vi "H2O_DIAL_NCAR_4CH_v4.04.vi"() -> ()   [LabVIEW 2012]
uses:
  C:/Users/H2ODial/Desktop/Shared Telescope WV DIAL Code/Libraries and VIs/PowerMeterCommands.dll
  Libraries and VIs/PowerMeterCommands.dll
  <vilib>/DAQmx/write.llb/DAQmx Write (Digital 1D Bool NChan 1Samp 1Line).vi
  <vilib>/DAQmx/miscellaneous.llb/DAQmx Fill In Error Info.vi
  <vilib>/Analysis/baseanly.llb/Mean (DBL).vi
  Libraries and VIs/Scalar_Data.vi
  Libraries and VIs/Scalar_Data_3.vi
  Libraries and VIs/Scalar_Data_2.vi
  Libraries and VIs/Scalar_Data_4.vi
  <vilib>/Analysis/NI_AALBase.lvlib
  Libraries and VIs/CLDevIFace.dll
panel:
  out "FileHour":i32=19
  out "L_Count":i32=64
  out "sigma_off_total":dbl[](array[numeric])=[5.235525125067343e-25, 5.206358319245337e-25, 5.177318750524933e-25, 5.148406424862825e-25, 5.119621341127451e-25, 5.090963491196627e-25, 5.062432860011865e-25, 5.034029425635027e-25, 5.005753159352157e-25, 4.977604025706667e-25, 4.949581982592347e-25, 4.921686981325722e-25, 4.893918966711095e-25, 4.866277877122191e-25, 4.8387636445644285e-25, 4.811376194764721e-25, 4.784115447230487e-25, 4.756981315339233e-25, 4.729973706394386e-25, 4.703092521721628e-25, 4.6763376567211625e-25, 4.6497090009594435e-25, 4.623206438225019e-25, 4.596829846622293e-25, 4.57057909862005e-25, 4.544454061150213e-25, 4.518454595652437e-25, 4.492580558158126e-25, 4.4668317993693425e-25, 4.441208164702635e-25, 4.41570949437918e-25, 4.390335623482575e-25, 4.365086382028137e-25, 4.339961595028071e-25, 4.314961082547237e-25, 4.290084659777996e-25, 4.2653321370993085e-25, 4.240703320135042e-25, 4.216198009811418e-25, 4.191816002426457e-25, 4.16755708969195e-25, 4.143421058805604e-25, 4.1194076924960845e-25, 4.095516769084665e-25, 4.0717480625238245e-25, 4.0481013424706545e-25, 4.0245763743206737e-25, 4.001172919260011e-25, 3.977890734322512e-25, 3.9547295724256756e-25, 3.931689182419048e-25, 3.908769309139365e-25, 3.8859696934393876e-25, 3.863290072236815e-25, 3.840730178557474e-25, 3.8182897415734565e-25, 3.7959684866403156e-25, 3.773766135338825e-25, 3.7516824055099053e-25, 3.729717011286995e-25, 3.707869663137923e-25, 3.686140067893342e-25, 3.664527928779591e-25, 3.643032945453827e-25, 3.621654814033011e-25, 3.600393227122229e-25, 3.579247873843723e-25, 3.5582184398664743e-25, 3.5373046074361216e-25, 3.5165060553938904e-25, 3.4958224592064764e-25, 3.475253490990589e-25, 3.454798819536632e-25, 3.4344581103303625e-25, 3.414231025576395e-25, 3.394117224218377e-25, 3.37411636196096e-25, 3.3542280912885406e-25, 3.3344520614845767e-25, 3.3147879186525413e-25, 3.295235305730259e-25, 3.275793862509532e-25, 3.2564632256504646e-25, 3.237243028702917e-25, 3.2181329021119735e-25, 3.1991324732434905e-25, 3.180241366390581e-25, 3.161459202790299e-25, 3.142785600633377e-25, 3.1242201750825597e-25, 3.1057625382770893e-25, 3.0874122993477767e-25, 3.0691690644282785e-25, 3.051032436660927e-25, 3.0330020162078266e-25, 3.0150774002602592e-25, 2.997258183045521e-25, 2.979543955833093e-25, 2.961934306943937e-25, 2.944428821752431e-25, 2.9270270826932477e-25, 2.909728669267514e-25, 2.8925331580414936e-25, 2.875440122654977e-25, 2.8584491338173137e-25, 2.841559759313169e-25, 2.8247715639976386e-25, 2.80808410980223e-25, 2.791496955724979e-25, 2.775009657833479e-25, 2.7586217692567447e-25, 2.742332840183121e-25, 2.7261424178518227e-25, 2.710050046547509e-25, 2.6940552675881075e-25, 2.6781576193155516e-25, 2.6623566370876434e-25, 2.646651853260364e-25, 2.6310427971768174e-25, 2.615528995144771e-25, 2.600109970428841e-25, 2.5847852432207883e-25, 2.569554330624564e-25, 2.554416746633416e-25, 2.5393720020962457e-25, 2.5244196047033826e-25, 2.5095590589459477e-25, 2.4947898660936654e-25, 2.480111524155541e-25, 2.4655235278440513e-25, 2.451025368544176e-25, 2.436616534266772e-25, 2.422296509605852e-25, 2.408064775697375e-25, 2.3939208101763006e-25, 2.3798640871112015e-25, 2.365894076971971e-25, 2.352010246556833e-25, 2.3382120589521406e-25, 2.324498973455175e-25, 2.3108704455300754e-25, 2.2973259267270024e-25, 2.283864864626908e-25, 2.270486702764721e-25, 2.257190880557015e-25, 2.2439768332388837e-25, 2.2308439917739663e-25, 2.2177917827749597e-25, 2.20481962844103e-25, 2.19192694645104e-25, 2.179113149897461e-25, 2.166377647190967e-25, 2.153719841983278e-25, 2.1411391330535246e-25, 2.1286349142540036e-25, 2.1162065743868337e-25, 2.103853497130775e-25, 2.091575060946101e-25, 2.079370638983031e-25, 2.0672395989815037e-25, 2.0551813031976677e-25, 2.0431951082869756e-25, 2.0312803652523447e-25, 2.019436419319984e-25, 2.0076626098781596e-25, 1.9959582703908636e-25, 1.9843227283026113e-25, 1.9727553050009988e-25, 1.9612553156963306e-25, 1.9498220693936616e-25, 1.9384548688025462e-25, 1.9271530103114487e-25, 1.915915783921294e-25, 1.9047424731896738e-25, 1.8936323552292957e-25, 1.8825847006561212e-25, 1.8715987735714719e-25, 1.8606738315918164e-25, 1.8498091257941087e-25, 1.8390039007904753e-25, 1.8282573946936752e-25, 1.8175688392200846e-25, 1.80693745969556e-25, 1.7963624751388698e-25, 1.7858430983630522e-25, 1.7753785360393623e-25, 1.7649679888396773e-25, 1.7546106515613228e-25, 1.7443057132789558e-25, 1.7340523575155863e-25, 1.723849762422857e-25, 1.7136971010131167e-25, 1.7035935413825008e-25, 1.6935382469544605e-25, 1.6835303767796407e-25, 1.6735690858143057e-25, 1.6636535252563445e-25, 1.653782842907513e-25, 1.643956183497921e-25, 1.6341726891478545e-25, 1.624431499756322e-25, 1.6147317534796005e-25, 1.6050725871551994e-25, 1.5954531368896971e-25, 1.585872538492723e-25, 1.576329928151117e-25, 1.566824442883223e-25, 1.5573552212546758e-25, 1.5479214039898043e-25, 1.5385221346219397e-25, 1.5291565602013113e-25, 1.519823831962039e-25, 1.5105231061650234e-25, 1.5012535447460145e-25, 1.49201431624485e-25, 1.482804596459418e-25, 1.4736235693849326e-25, 1.46447042805166e-25, 1.455344375360034e-25, 1.4462446250285657e-25, 1.4371704024629248e-25, 1.4281209456557682e-25, 1.4190955061389853e-25, 1.410093350012645e-25, 1.4011137586880333e-25, 1.3921560301221658e-25, 1.3832194795253431e-25, 1.3743034404767374e-25, 1.3654072658699072e-25, 1.3565303288298996e-25, 1.3476720236918642e-25, 1.3388317669734332e-25, 1.3300089982893968e-25, 1.3212031812258562e-25, 1.3124138043688156e-25, 1.3036403820696332e-25, 1.2948824553577423e-25, 1.2861395928315612e-25, 1.2774113913410786e-25, 1.2686974768684636e-25, 1.2599975053009544e-25, 1.2513111630057894e-25, 1.2426381676023619e-25, 1.2339782685325752e-25, 1.2253312476934588e-25, 1.2166969199403071e-25, 1.2080751335374065e-25, 1.1994657705541538e-25, 1.1908687474046665e-25, 1.182284014933639e-25, 1.1737115587808914e-25, 1.1651513996305814e-25, 1.1566035931942852e-25, 1.1480682304187532e-25, 1.1395454373665928e-25, 1.1310353751750977e-25, 1.1225382399779688e-25, 1.1140542626706877e-25, 1.1055837085176348e-25, 1.097126877076807e-25, 1.0886841014622313e-25, 1.0802557481625692e-25, 1.07184221622742e-25, 1.0634439369229237e-25, 1.0550613727868173e-25, 1.0466950171251473e-25, 1.038345393031225e-25, 1.0300130526116006e-25, 1.0216985760646603e-25, 1.0134025706453978e-25, 1.0051256696943142e-25, 9.968685315566847e-26, 9.886318383691271e-26, 9.804162950309608e-26, 9.722226278487634e-26, 9.640515833439737e-26, 9.559039270504641e-26]
  out "sigma_on_total":dbl[](array[numeric])=[2.797932674537263e-23, 2.7919260210529697e-23, 2.7857624681005274e-23, 2.7794434391305526e-23, 2.772970398522555e-23, 2.766344851030676e-23, 2.75956834067003e-23, 2.752642449576685e-23, 2.7455687974466073e-23, 2.738349040027496e-23, 2.730984868354913e-23, 2.723478007699131e-23, 2.715830216384083e-23, 2.708043284811922e-23, 2.700119034195852e-23, 2.6920593156696255e-23, 2.683866008939376e-23, 2.675541021372197e-23, 2.6670862865706313e-23, 2.6585037635576785e-23, 2.649795435279164e-23, 2.6409633077211456e-23, 2.632009408457337e-23, 2.622935785817294e-23, 2.613744507314058e-23, 2.6044376589247666e-23, 2.5950173434598757e-23, 2.5854856796179397e-23, 2.5758448009875033e-23, 2.5660968544222956e-23, 2.556243999280564e-23, 2.5462884060976083e-23, 2.5362322554945982e-23, 2.5260777370381022e-23, 2.5158270479358892e-23, 2.505482392145547e-23, 2.4950459792064817e-23, 2.484520023083591e-23, 2.4739067410236316e-23, 2.4632083527131388e-23, 2.452427078874796e-23, 2.4415651405700084e-23, 2.4306247579414987e-23, 2.419608149375398e-23, 2.4085175301631292e-23, 2.397355112043402e-23, 2.3861231018430063e-23, 2.3748237005968667e-23, 2.3634591028590494e-23, 2.352031495518178e-23, 2.3405430569776974e-23, 2.3289959565846446e-23, 2.3173923533947887e-23, 2.3057343955308516e-23, 2.2940242194478666e-23, 2.282263949107109e-23, 2.2704556951731608e-23, 2.258601554403489e-23, 2.2467036088909498e-23, 2.2347639252740327e-23, 2.2227845543076132e-23, 2.2107675300632033e-23, 2.1987148693219933e-23, 2.18662857110243e-23, 2.1745106160433166e-23, 2.162362965811164e-23, 2.1501875625868626e-23, 2.137986328630551e-23, 2.1257611659233766e-23, 2.113513955448302e-23, 2.1012465569339107e-23, 2.0889608084552326e-23, 2.076658526056973e-23, 2.0643415033451598e-23, 2.0520115112091644e-23, 2.0396702974574623e-23, 2.0273195865824679e-23, 2.014961079439288e-23, 2.0025964529993626e-23, 1.9902273602298353e-23, 1.9778554297286174e-23, 1.9654822656439602e-23, 1.9531094474030767e-23, 1.9407385298246202e-23, 1.9283710425220375e-23, 1.916008490311647e-23, 1.9036523527571788e-23, 1.891304084249504e-23, 1.878965113795808e-23, 1.8666368452826158e-23, 1.854320657095235e-23, 1.842017902311335e-23, 1.829729908755202e-23, 1.81745797881863e-23, 1.8052033895967212e-23, 1.7929673929858462e-23, 1.7807512156964232e-23, 1.7685560592802502e-23, 1.756383100364305e-23, 1.744233490557376e-23, 1.732108356659952e-23, 1.7200088008822495e-23, 1.7079359007408066e-23, 1.6958907094876615e-23, 1.6838742559821464e-23, 1.6718875450901883e-23, 1.65993155762526e-23, 1.6480072508541525e-23, 1.6361155583187127e-23, 1.6242573903102193e-23, 1.6124336338929427e-23, 1.600645153253371e-23, 1.5888927898296925e-23, 1.5771773626269717e-23, 1.5654996683162563e-23, 1.553860481518072e-23, 1.5422605551758425e-23, 1.5307006206288193e-23, 1.519181387994595e-23, 1.50770354621203e-23, 1.4962677636431785e-23, 1.4848746879968784e-23, 1.4735249468084555e-23, 1.462219147707836e-23, 1.4509578784447202e-23, 1.439741707535912e-23, 1.4285711842133102e-23, 1.4174468389483338e-23, 1.4063691835697543e-23, 1.3953387115476105e-23, 1.3843558984350844e-23, 1.3734212019927912e-23, 1.3625350624750627e-23, 1.3516979029933517e-23, 1.340910129876358e-23, 1.3301721326484853e-23, 1.3194842846972786e-23, 1.308846943215553e-23, 1.298260449786731e-23, 1.2877251303686642e-23, 1.2772412958726839e-23, 1.2668092421859013e-23, 1.2564292506343541e-23, 1.2461015881516254e-23, 1.2358265075568203e-23, 1.2256042479710005e-23, 1.2154350349122617e-23, 1.2053190805695919e-23, 1.195256584279949e-23, 1.1852477325180829e-23, 1.1752926993686362e-23, 1.1653916466854379e-23, 1.1555447244520414e-23, 1.1457520708062173e-23, 1.1360138126272996e-23, 1.1263300654904525e-23, 1.1167009340815523e-23, 1.1071265124104599e-23, 1.0976068840545527e-23, 1.0881421223367986e-23, 1.0787322906900863e-23, 1.0693774427047456e-23, 1.0600776226092928e-23, 1.0508328652518817e-23, 1.0416431964807624e-23, 1.032508633335529e-23, 1.0234291841778234e-23, 1.014404849115549e-23, 1.0054356199498731e-23, 9.965214805919994e-24, 9.876624071246281e-24, 9.788583681497812e-24, 9.701093249022246e-24, 9.61415231391845e-24, 9.527760347380011e-24, 9.441916752482458e-24, 9.356620866076204e-24, 9.27187196198394e-24, 9.1876692506485e-24, 9.104011883065926e-24, 9.020898950407833e-24, 8.938329487852217e-24, 8.856302474691644e-24, 8.77481683652038e-24, 8.69387144736208e-24, 8.613465130247208e-24, 8.533596659539215e-24, 8.454264762212557e-24, 8.375468119356111e-24, 8.297205367646391e-24, 8.219475100553976e-24, 8.14227587023874e-24, 8.065606188690859e-24, 7.9894645288563e-24, 7.913849326432266e-24, 7.838758980703018e-24, 7.764191856046392e-24, 7.69014628339956e-24, 7.61662056058579e-24, 7.543612954624664e-24, 7.471121702227356e-24, 7.399145011371256e-24, 7.327681061555103e-24, 7.256728006172217e-24, 7.18628397208889e-24, 7.116347062363852e-24, 7.046915355389474e-24, 6.977986907338961e-24, 6.909559752711582e-24, 6.84163190507593e-24, 6.774201358193111e-24, 6.707266086331618e-24, 6.640824046318606e-24, 6.5748731770349155e-24, 6.509411401784767e-24, 6.444436627394219e-24, 6.37994674615007e-24, 6.315939636375851e-24, 6.252413162819167e-24, 6.189365177933176e-24, 6.126793522223083e-24, 6.064696024770319e-24, 6.003070504094802e-24, 5.9419147695012916e-24, 5.8812266199939874e-24, 5.821003847135055e-24, 5.761244233601571e-24, 5.7019455549703875e-24, 5.6431055801137746e-24, 5.584722071428577e-24, 5.526792785547098e-24, 5.469315474021976e-24, 5.41228788367443e-24, 5.3557077567834e-24, 5.299572832346729e-24, 5.243880845770717e-24, 5.188629529638899e-24, 5.133816614447439e-24, 5.079439828285976e-24, 5.0254968978526986e-24, 4.971985548989939e-24, 4.918903506350013e-24, 4.866248494353352e-24, 4.814018237267727e-24, 4.762210459841147e-24, 4.710822887499211e-24, 4.6598532465403046e-24, 4.609299264328646e-24, 4.559158670401048e-24, 4.5094291956991564e-24, 4.460108573396636e-24, 4.4111945394283046e-24, 4.362684832116821e-24, 4.3145771930692756e-24, 4.266869366921456e-24, 4.219559101711097e-24, 4.1726441493533976e-24, 4.1261222657367405e-24, 4.0799912104676045e-24, 4.034248748141451e-24, 3.988892647248926e-24, 3.9439206815329655e-24, 3.899330629138496e-24, 3.8551202738110765e-24, 3.811287404055379e-24, 3.7678298141883e-24, 3.7247453038325186e-24, 3.682031678396438e-24, 3.639686749212774e-24, 3.597708333465123e-24, 3.5560942545295516e-24, 3.514842342094612e-24, 3.473950431977779e-24, 3.4334163667422104e-24, 3.393237995303275e-24, 3.353413173235189e-24, 3.313939763152937e-24]
  out "background start":u32=269
  in  "Tab Control 2":enum32{"WV ND far", "WV ND near"}(tab)
  out "Water Vapor Number Density":dbl[][](graph)=[[2.0850030204725254, 1.6437816356735586, 1.585155342040526, 1.4766994515960457, 1.30036312748755, 1.2199808815388116, 1.2370910084987519, 1.215025732560631, 1.2094080739137962, 1.241574717944049, 1.2400023005883922, 1.27849779833147, 1.1795592586311967, 1.0177397521499008, 0.9252100877503859, 0.7984582340031915, 0.7980739516878171, 0.981563170106793, 1.1781709472616928, 1.2604407853067179, 1.2878310718082464, 0.9634305882669428, 0.6969286050839552, 1.1038803104348858, 1.3635527853492146, 1.2756168466381246, 1.126651831817223, 0.8778144411805149, 1.0190755684005814, 0.7047223129802344, -0.11061275401062327, 0.32290982101144, 0.00359197927144264, -0.7090099831195374, 0.893795498062288, 1.3190587788482702, 0.5035252151885548, 0.28968410009682993, 0.18512581697537367, 0.3528560626576347, 3.2334978562537446, 2.5390776007956823, -0.7673398002393842, -0.394060585705837, 0.1936892729399504, -0.00042004503324332, 0.6488032887854288, -1.7199954662418278, -2.7250956673421256, -2.829602242413674, -2.8562819886715487, 0.24819172415081983, 2.4357247968367557, -0.08684114825213345, 0.33472910263403344, 1.4525262638352578, 0.6864828027636564, -0.8773873676446362, -0.7748026661236419, -0.8964337587498109, -1.3574906833153229, -1.9055460673602915, -1.8292121536809087, -2.635674405161918, -4.437757131889345, -5.4711270091092965, -4.930064996443606, -2.073930252529242, -0.56696116876414, 3.0237519462406395, 4.188864159369365, -1.179054090698212, -2.0895392573583993, 1.096562317594488, 3.8376615661152935, 3.813963625998703, 4.150238128596571, 1.2755121222242172, 1.722039359608823, -5.434206523456943, -5.690067282284008, 0.05770429680683136, 0.2219851428874463, 7.0959946213841985, 1.532667826481585, -0.5776567177838131, -3.1758034812173244, 3.496673290983224, 0.04729286306369408, 0.19208777119169312, 4.302023971326133, 0.01865185774192832, 1.2460870798892005, -2.484809490618561, -0.6929405246784887, 1.5500192808793258, -0.05367189562925824, -5.735849575728608, -10.29033614959377, -6.410256857872558, -5.005499582994593, -4.426020458002386, 3.8865322258423878, -8.339098819142706, -9.85784046414273, -9.45196269897021, -5.509570293351291, -1.1199600054419636, 6.7032461962178616, -4.1633235794603864, 2.0683846017602328, 3.572831455646544, -13.574834245937282, -1.354642132743935, 4.298010924764007, -4.7498368773700355, 5.349703968676538, 9.152156484607096, 8.23822238004354, 11.236456605215093, 4.6977921044492374, -8.712287895980495, -7.563029666917176, 11.007974192105422, 12.165531573107202, 11.594288918432497, 3.370534175609367, -35.26246376101609, -17.948505635707626, -2.8000376045066497, -1.5924615735558247, 10.16969778493625, 5.877930799567327, -24.882484593161845, -9.516571042712105, -1.6853765938446423, -12.119319412457292, 28.525305472061554, 13.695570360112042, 10.944237189694553, -4.978227526265883, -0.44379160486049024, 12.331720846487988, 14.911137981786128, 3.216797260224393, 3.8658670134448565, 11.945343806227195, -0.5474095512917645, -2.9509077491873588, -28.863902827765653, -4.294981423276254, 0.1988682777637764, -13.211149394496491, 5.808378000312744, 16.358090642229662, -1.4997757775899234, -20.411277889358345, 2.898487754529748, -0.6745628910628864, 16.536306010274835, 0.6145433580451252, -3.6722274359744307, 18.913701367295182, 12.528730096566148, -28.431881689114736, -4.669563197294236, 28.61360237595095, -14.608108405047787, -18.932456658706972, 8.510895794846949, 4.367610244303744, -7.896210598721369, -33.65782516306702, -15.516623535496258, 15.753404769314882, -0.8897774586406809, 9.708498007840978, 24.13002108358846, -15.620252851147146, -15.249309427554964, -8.17893430618913, -8.132812569975494, 24.140582206511233, -2.1172348165747623, -14.222694350100634, -3.0031622935380584, -28.73267843976295, -12.340614051377894, 27.52998202950442, -15.558704125250053, 24.126926460529376, 25.711179733884677, -40.04430966856323, -6.274211048141865, -4.540478314335458, 8.688842305429981, 3.76326811922837, -6.656379689914578, -17.935547234154576, 15.474596374301731, -4.549990267263325, -16.996817668296618, 40.451771082531295, 24.3573227243969, 13.31160725295816, 26.040765428929117, 15.968201995244634, 24.26538927457644, -23.10849151042884, 11.31205185038729, -6.111927224105964, 7.201296036063291, 4.320464599920811, 21.56516811072391, 10.036241250128949, -22.846017259183665, 9.584823226618145, -29.59233799457406, 55.86100537533308, 8.326728755523506, -10.071822516636537, -12.516373180368932, 33.53909345931459, -23.202570298285117, 1.3605784639618446, -3.939394952264914, 16.055757489219552, 25.387570363295236, 0.40448320363909185, 35.00096495746182, 15.660340156158572, -3.805076154606008, -34.56927048910243, -14.259486007723957, -17.820859719934365, -33.61661057208902, -58.732906499454884, -3.6372704024162408, 11.610203197310321, 1.8116853683437568, -5.123600805072583, 14.543741009244814, -7.16832268645471, 77.44415327164283, -53.0182416582464, -21.01003828902848, 7.838641860670423, -23.503259151305624, -22.51128145040154, -49.73789705224452, -3.7742787786248075, 33.15558831364227, 44.026419860724644, -86.50170167029069, 50.055327704940204, 48.860804186022065, 5.656765694967322, -8.84047801247566, 10.232888014228477, -49.490816604374494, -27.733700249649516, -50.55140951741612, -64.0940844805227, 0.9991234230215273, -2.510153727691791, -38.72495478502656, -32.93879155638287, 22.12815841351247, -31.9911923562734, 61.47922701145286, 16.31717375874161, 11.0359028192536, 15.334090958525035, -0.607939340584462, 0.7152432696449843, 34.35519313891373, 0.0, 0.0, 0.0, 0.0]]
  out "Water Vapor Number Density 2":dbl[][](graph)=[[nan, nan, nan, nan, nan, nan, nan, nan, nan, nan, nan, nan, nan, nan, nan, nan, nan, nan, nan, nan, nan, nan, nan, nan, nan, nan, nan, nan, nan, nan, nan, nan, nan, nan, nan, nan, nan, nan, nan, nan, nan, nan, nan, nan, nan, nan, nan, nan, nan, nan, nan, nan, nan, nan, nan, nan, nan, nan, nan, nan, nan, nan, nan, nan, nan, nan, nan, nan, nan, nan, nan, nan, nan, nan, nan, nan, nan, nan, nan, nan, nan, nan, nan, nan, nan, nan, nan, nan, nan, nan, nan, nan, nan, nan, nan, nan, nan, nan, nan, nan, nan, nan, nan, nan, nan, nan, nan, nan, nan, nan, nan, nan, nan, nan, nan, nan, nan, nan, nan, nan, nan, nan, nan, nan, nan, nan, nan, nan, nan, nan, nan, nan, nan, nan, nan, nan, nan, nan, nan, nan, nan, nan, nan, nan, nan, nan, nan, nan, nan, nan, nan, nan, nan, nan, nan, nan, nan, nan, nan, nan, nan, nan, nan, nan, nan, nan, nan, nan, nan, nan, nan, nan, nan, nan, nan, nan, nan, nan, nan, nan, nan, nan, nan, nan, nan, nan, nan, nan, nan, nan, nan, nan, nan, nan, nan, nan, nan, nan, nan, nan, nan, nan, nan, nan, nan, nan, nan, nan, nan, nan, nan, nan, nan, nan, nan, nan, nan, nan, nan, nan, nan, nan, nan, nan, nan, nan, nan, nan, nan, nan, nan, nan, nan, nan, nan, nan, nan, nan, nan, nan, nan, nan, nan, nan, nan, nan, nan, nan, nan, nan, nan, nan, nan, nan, nan, nan, nan, nan, nan, nan, nan, nan, nan, nan, nan, nan, nan, nan, nan, nan, nan, nan, nan, nan, nan, nan, 0.0, 0.0, 0.0, 0.0]] caption="Water Vapor Number Density"
  out "RingBuffer offline near":dbl[][](array[numeric])
  out "RingBuffer aerosol near":dbl[][](array[numeric])
  in  "?":T1(tab)=enum."Raw Counts far"
  out "NRB":dbl[][](graph)=[[0.005926456667752352, 0.00034845887869832493, 0.00117345593822808, 0.002732380746740355, 0.005084886684210653, 0.008132850694616053, 0.0116541750651601, 0.015219667698509734, 0.018606332351052295, 0.0218004400758057, 0.024507078478819787, 0.02689031435072529, 0.02929831081577581, 0.0315427037929839, 0.03335112978817941, 0.03525413620901254, 0.03728758615178838, 0.03878274790840357, 0.03887699584826217, 0.03674294955920922, 0.033802343966385755, 0.03268171593006662, 0.034202254837176274, 0.03616439929082925, 0.03682729838732918, 0.03583520192541121, 0.0336166963339548, 0.03144028501113685, 0.02903704288238401, 0.026445123328020622, 0.02431657360774544, 0.022683557967303855, 0.021610770611037458, 0.020428065925194538, 0.01933597330300677, 0.018269668608962168, 0.01760669738842388, 0.01729134198515122, 0.016360408778451793, 0.016435295905221137, 0.017096235707125273, 0.01732741053273295, 0.017684084999968628, 0.017856021895490994, 0.016659339456252698, 0.014142438147388029, 0.012118368226233222, 0.010323788633718637, 0.008334493517991313, 0.008443265914553294, 0.00839675379113525, 0.007583456336000032, 0.008149114133626848, 0.008346168279196766, 0.008078002538559965, 0.00788068110930718, 0.008309895111598447, 0.007594904462158592, 0.006309684597299873, 0.0063621222028002414, 0.005633381728465795, 0.005964037138631247, 0.006893384939459379, 0.005665084378278788, 0.006806987647958848, 0.007432890551790987, 0.004751652260563181, 0.0048556087855860155, 0.005785976896777462, 0.005869192731966311, 0.004908143097055829, 0.00425145518138192, 0.006124122691864267, 0.004962740164068838, 0.0051269265586496235, 0.005174752348916562, 0.0029343245128427265, 0.004682132358603469, 0.005466013949020874, 0.002935255717246242, 0.0030728489507631795, 0.005405527925092298, 0.005109745084060786, 0.0035469393249789823, 0.003168537758727533, 0.00383283939731712, 0.005403276416428827, 0.006049937560898696, 0.006280581727541977, 0.007115159077609801, 0.006528474699620713, 0.004967510133987116, 0.0030254536405443723, 0.004619160493057294, 0.005156445579642906, 0.0041431865870912325, 0.003205973312806835, 0.003627037361616739, 0.0068569500535467474, 0.00663339984399211, 0.0033106318284078003, 0.001125494867474759, 0.002961974770465925, 0.006677209621225703, 0.006006324358505338, -2.9113641335633503e-05, -0.0011569518147719314, 0.0030978527449643163, 0.0034787346198737537, 1.5676179877085825e-05, 0.0006145573082985116, 0.003664733892477403, 0.003912443955116488, 0.0052027132407723685, 0.004172101822527913, 0.0006101542570013053, 0.0033785144395073697, 0.003959663306511802, 0.0009356643379633596, -0.0008488436888549461, -0.0003603950068261491, 0.0009352276162559068, -0.00041160808513453456, 0.0008665396489930335, 0.003502069950398978, 0.0023859234245020462, -0.000605981884669559, 0.00270637392787425, 0.005357549317683901, -0.004422709702591833, -0.00190091042773388, 0.0034312287433246364, -0.0005041738540758441, 0.0021285681932495756, 7.083431590314749e-05, 0.0028036327356922033, 0.00689374696561347, 0.003972303927274524, 0.0004755963019097945, -0.001434690128721588, 0.003348415241044566, 0.006021540097100841, 0.0045435452046482154, 0.005050586968564978, 0.0011031809981202107, -0.0013531799341342163, -0.0013577824057589966, -0.004895122284460349, -0.003437103690692682, 0.0006850239376734047, 0.0033823361669823894, -0.0002993241786557989, -0.0017135031236348802, -0.0024272897633639515, -0.0014162131683847245, -0.0004256351746895539, -0.0019000708485824003, 0.005530557693975901, 0.0084339698807476, 0.004709624787800002, -0.0035764638573479272, -0.0019380209375184376, 0.0066434190765325436, -0.0023171956809975654, -0.006948396385216679, -0.00012495078483892955, -0.005329378099251803, -0.004333004380050942, 0.0031267045111360134, -0.0013853311217609417, -0.0035041827316570364, -0.0004407672565580389, -0.0013958821485772152, 0.0033929024277816835, 0.007479050805328789, 0.00437430538852055, 0.004850337256527115, 0.004782151852909807, 0.005894573743199213, 0.00984346293300644, 0.01237248760973823, 0.01027799631704262, 0.0024079709356714003, 0.0007895204735910104, 0.003946301707784646, 0.004190775740572, 0.0035337383805607173, 0.0015568623503716252, 0.007034373389594776, 0.0026658650988290776, 0.0019850516126564896, 0.00785645917750268, 0.000530838475279584, 0.003876387634669509, -0.007487973194147328, -0.004230425259091719, 0.011061521406492938, 0.006475871793724494, 0.009748074027175178, -0.0011659954493232437, 0.003820950765333305, 0.004916347793299921, -0.0017351201798288354, 0.005930759433534724, -0.0006533464675369102, 0.0033261819655687956, -0.00352507086236981, -0.0032509345134268293, -0.0013581824884157324, -0.009169906507551565, -0.01061288585730394, -0.010218797455319647, 0.002821346039036585, 0.012637661706030909, 0.014313141794587331, -0.00024178104507830393, -0.0053380227866509965, -0.009574029762005911, -0.012209595231276224, 0.0013481528825468932, -0.005410079028084043, -0.009162405514005137, -0.002802546729563259, 0.008255766922838005, 0.009969350041942705, -0.00036394377149788124, -0.0001001377400367479, -0.009091913816734288, -0.010360775600521087, -0.001953236110965131, 0.004078797338320419, 0.0011157095574698026, -0.019200974575226553, -0.005781524354338799, 0.0023252767695942506, -0.010210150631123164, 0.0006185440763654871, 0.0014677064390170292, -0.0108043902235317, -0.0077608333698953366, 0.004665326006792024, 0.006107778031363839, -0.0029835349786772962, -0.017547322075334913, -0.010498271138224758, -0.009682539447614396, 0.005374761218746404, 0.007091697304180774, -0.02273179292127545, -0.014736766744659825, 0.010121076962341406, 0.0069932127456768, -0.012480415550388788, -0.009570292753878974, 0.003327615811897804, -0.011462135732023291, -0.018654033185619246, -0.008149368712937241, -0.007647774814481756, -0.012523750403639214, -0.019327474639449553, -0.03188149127146276, -0.009812462957050768, 0.01801399465388992, -0.003047829418398536, 0.0002750042719365171, 0.0003694344987373863, 0.002372822109574436, 0.0014062126414341747, -0.01605563624828103, -0.01836311908670994, -0.006038538007938858, 0.0088832116573971, 0.0010699140747426792, 0.006907341304357512, 0.02393261407692816, 0.017793910000995054, 0.0, 0.0, 0.0]] caption="Water Vapor Number Density"
  out "NRB 2":dbl[][](graph) caption="Water Vapor Number Density"
  out "raw counts":dbl[][](graph)=[[50996.6, 384.6, 639.6, 801.6, 986.6, 1158.6, 1285.6, 1289.6, 1247.6, 1114.6, 1093.6, 1009.6, 970.6, 934.6, 819.6, 813.6, 705.6, 741.6, 656.6, 514.6, 463.6, 355.6, 347.6, 339.6, 316.6, 265.6, 244.6, 189.6, 161.6, 143.6, 136.6, 159.6, 119.6, 117.6, 77.6, 94.6, 87.6, 82.6, 61.599999999999994, 57.599999999999994, 46.599999999999994, 42.599999999999994, 37.599999999999994, 43.599999999999994, 53.599999999999994, 34.599999999999994, 19.599999999999994, 29.599999999999994, 3.5999999999999943, 14.599999999999994, 27.599999999999994, 28.599999999999994, 12.599999999999994, 0.5999999999999943, 17.599999999999994, 2.5999999999999943, -15.400000000000006, 38.599999999999994, 9.599999999999994, 4.599999999999994, 30.599999999999994, -15.400000000000006, 28.599999999999994, 1.5999999999999943, -19.400000000000006, 50.599999999999994, 5.599999999999994, 32.599999999999994, 5.599999999999994, 28.599999999999994, -21.400000000000006, 39.599999999999994, -26.400000000000006, -14.400000000000006, 2.5999999999999943, 15.599999999999994, 4.599999999999994, -10.400000000000006, -10.400000000000006, -7.400000000000006, -30.400000000000006, 7.599999999999994, 12.599999999999994, 0.5999999999999943, -8.400000000000006, -8.400000000000006, 1.5999999999999943, 2.5999999999999943, 3.5999999999999943, 19.599999999999994, 12.599999999999994, 15.599999999999994, -0.4000000000000057, 13.599999999999994, 14.599999999999994, 17.599999999999994, -8.400000000000006, -19.400000000000006, 23.599999999999994, 16.599999999999994, 1.5999999999999943, 14.599999999999994, 18.599999999999994, -3.4000000000000057, 16.599999999999994, 5.599999999999994, -17.400000000000006, -15.400000000000006, -4.400000000000006, -2.4000000000000057, -18.400000000000006, -4.400000000000006, 1.5999999999999943, 0.5999999999999943, 15.599999999999994, -14.400000000000006, -4.400000000000006, 8.599999999999994, -10.400000000000006, -16.400000000000006, 17.599999999999994, -23.400000000000006, 0.5999999999999943, -12.400000000000006, -19.400000000000006, 10.599999999999994, 1.5999999999999943, 6.599999999999994, -25.400000000000006, 5.599999999999994, 7.599999999999994, 16.599999999999994, 6.599999999999994, 0.5999999999999943, 17.599999999999994, -7.400000000000006, 27.599999999999994, 17.599999999999994, 13.599999999999994, 15.599999999999994, -15.400000000000006, -2.4000000000000057, -11.400000000000006, -10.400000000000006, 3.5999999999999943, -6.400000000000006, 13.599999999999994, -8.400000000000006, -28.400000000000006, 3.5999999999999943, -14.400000000000006, -15.400000000000006, -4.400000000000006, 31.599999999999994, -19.400000000000006, 3.5999999999999943, -0.4000000000000057, 11.599999999999994, -14.400000000000006, 12.599999999999994, -14.400000000000006, 28.599999999999994, 14.599999999999994, 4.599999999999994, -10.400000000000006, 19.599999999999994, 17.599999999999994, -28.400000000000006, -16.400000000000006, 17.599999999999994, 1.5999999999999943, -18.400000000000006, 5.599999999999994, -18.400000000000006, -20.400000000000006, -29.400000000000006, 16.599999999999994, 0.5999999999999943, -33.400000000000006, -5.400000000000006, 16.599999999999994, 7.599999999999994, -1.4000000000000057, 5.599999999999994, -7.400000000000006, 25.599999999999994, 1.5999999999999943, 15.599999999999994, -0.4000000000000057, 15.599999999999994, 20.599999999999994, -15.400000000000006, -4.400000000000006, -25.400000000000006, -0.4000000000000057, -28.400000000000006, 6.599999999999994, -16.400000000000006, 3.5999999999999943, 22.599999999999994, -10.400000000000006, 11.599999999999994, 9.599999999999994, -26.400000000000006, -9.400000000000006, -22.400000000000006, -1.4000000000000057, 3.5999999999999943, 21.599999999999994, -36.400000000000006, -4.400000000000006, -4.400000000000006, -25.400000000000006, -12.400000000000006, -12.400000000000006, 23.599999999999994, -7.400000000000006, 10.599999999999994, 0.5999999999999943, 5.599999999999994, 15.599999999999994, 1.5999999999999943, 1.5999999999999943, 3.5999999999999943, 0.5999999999999943, -4.400000000000006, -10.400000000000006, -46.400000000000006, 19.599999999999994, -13.400000000000006, -5.400000000000006, -0.4000000000000057, -11.400000000000006, -3.4000000000000057, -9.400000000000006, -5.400000000000006, -21.400000000000006, -10.400000000000006, -0.4000000000000057, -16.400000000000006, -14.400000000000006, 3.5999999999999943, 2.5999999999999943, -9.400000000000006, 12.599999999999994, -2.4000000000000057, 19.599999999999994, 10.599999999999994, -24.400000000000006, 0.5999999999999943, -2.4000000000000057, 2.5999999999999943, -26.400000000000006, 0.5999999999999943, 22.599999999999994, 2.5999999999999943, -27.400000000000006, -17.400000000000006, -14.400000000000006, -9.400000000000006, -23.400000000000006, -33.400000000000006, -2.4000000000000057, -30.400000000000006, 16.599999999999994, -5.400000000000006, 3.5999999999999943, 3.5999999999999943, -22.400000000000006, -7.400000000000006, -6.400000000000006, 21.599999999999994, -4.400000000000006, -0.4000000000000057, -9.400000000000006, 13.599999999999994, 23.599999999999994, -10.400000000000006, -20.400000000000006, 0.0]] caption="Water Vapor Number Density"
  out "raw counts near":dbl[][](graph) caption="Water Vapor Number Density"
  out "Aerosol Smoothed 2":dbl[](array[numeric])
  out "Off-Line Smoothed 2":dbl[](array[numeric])
  out "Off-Line Bin Readings 2":dbl[](array[numeric])
  out "On-Line Smoothed 2":dbl[](array[numeric])
  out "On-Line Bin Readings 2":dbl[](array[numeric])
  in  "stop":bool
  in  "Reset Average":bool=TRUE
  in  "Save Data?":bool=TRUE
  in  "Collect Data?":bool=TRUE
  in  "ILX Address":i32=6 min=0 step=1
  in  "Lambda On DBR Current":dbl=171.04999999999876
  in  "Lambda Off DBR Current":dbl=172.9599999999997
  in  "Tab Control":T2(tab)=enum."g/m^3"
  out "Water Vapor Number Density  2":cluster{"Y":dbl[], "Y":dbl[]}[](graph)=[{"Y"=array[276 elements], "Y"=array[280 elements]}, {"Y"=[nan, nan, nan, nan, nan, nan, nan, nan, nan, nan, nan, nan, nan, nan, nan, nan, nan, nan, nan, nan, nan, nan, nan, nan, nan, nan, nan, nan, nan, nan, nan, nan, nan, nan, nan, nan, nan, nan, nan, nan, nan, nan, nan, nan, nan, nan, nan, nan, nan, nan, nan, nan, nan, nan, nan, nan, nan, nan, nan, nan, nan, nan, nan, nan, nan, nan, nan, nan, nan, nan, nan, nan, nan, nan, nan, nan, nan, nan, nan, nan, nan, nan, nan, nan, nan, nan, nan, nan, nan, nan, nan, nan, nan, nan, nan, nan, nan, nan, nan, nan, nan, nan, nan, nan, nan, nan, nan, nan, nan, nan, nan, nan, nan, nan, nan, nan, nan, nan, nan, nan, nan, nan, nan, nan, nan, nan, nan, nan, nan, nan, nan, nan, nan, nan, nan, nan, nan, nan, nan, nan, nan, nan, nan, nan, nan, nan, nan, nan, nan, nan, nan, nan, nan, nan, nan, nan, nan, nan, nan, nan, nan, nan, nan, nan, nan, nan, nan, nan, nan, nan, nan, nan, nan, nan, nan, nan, nan, nan, nan, nan, nan, nan, nan, nan, nan, nan, nan, nan, nan, nan, nan, nan, nan, nan, nan, nan, nan, nan, nan, nan, nan, nan, nan, nan, nan, nan, nan, nan, nan, nan, nan, nan, nan, nan, nan, nan, nan, nan, nan, nan, nan, nan, nan, nan, nan, nan, nan, nan, nan, nan, nan, nan, nan, nan, nan, nan, nan, nan, nan, nan, nan, nan, nan, nan, nan, nan, nan, nan, nan, nan, nan, nan, nan, nan, nan, nan, nan, nan, nan, nan, nan, nan, nan, nan, nan, nan, nan, nan, nan, nan, nan, nan, nan, nan, nan, nan], "Y"=array[280 elements]}]
  out "Absolute Humidity":cluster{"Y":dbl[], "Y":dbl[]}[](graph)=[{"Y"=array[276 elements], "Y"=array[280 elements]}, {"Y"=[nan, nan, nan, nan, nan, nan, nan, nan, nan, nan, nan, nan, nan, nan, nan, nan, nan, nan, nan, nan, nan, nan, nan, nan, nan, nan, nan, nan, nan, nan, nan, nan, nan, nan, nan, nan, nan, nan, nan, nan, nan, nan, nan, nan, nan, nan, nan, nan, nan, nan, nan, nan, nan, nan, nan, nan, nan, nan, nan, nan, nan, nan, nan, nan, nan, nan, nan, nan, nan, nan, nan, nan, nan, nan, nan, nan, nan, nan, nan, nan, nan, nan, nan, nan, nan, nan, nan, nan, nan, nan, nan, nan, nan, nan, nan, nan, nan, nan, nan, nan, nan, nan, nan, nan, nan, nan, nan, nan, nan, nan, nan, nan, nan, nan, nan, nan, nan, nan, nan, nan, nan, nan, nan, nan, nan, nan, nan, nan, nan, nan, nan, nan, nan, nan, nan, nan, nan, nan, nan, nan, nan, nan, nan, nan, nan, nan, nan, nan, nan, nan, nan, nan, nan, nan, nan, nan, nan, nan, nan, nan, nan, nan, nan, nan, nan, nan, nan, nan, nan, nan, nan, nan, nan, nan, nan, nan, nan, nan, nan, nan, nan, nan, nan, nan, nan, nan, nan, nan, nan, nan, nan, nan, nan, nan, nan, nan, nan, nan, nan, nan, nan, nan, nan, nan, nan, nan, nan, nan, nan, nan, nan, nan, nan, nan, nan, nan, nan, nan, nan, nan, nan, nan, nan, nan, nan, nan, nan, nan, nan, nan, nan, nan, nan, nan, nan, nan, nan, nan, nan, nan, nan, nan, nan, nan, nan, nan, nan, nan, nan, nan, nan, nan, nan, nan, nan, nan, nan, nan, nan, nan, nan, nan, nan, nan, nan, nan, nan, nan, nan, nan, nan, nan, nan, nan, nan, nan], "Y"=array[280 elements]}]
  out "NRB plot":cluster{"Y":dbl[], "Y":dbl[]}[](graph)
  in  "background length":i32=10
  out "Correction":cluster{"Y":dbl[], "Y":dbl[]}[](graph)=[{"Y"=array[277 elements], "Y"=array[280 elements]}, {"Y"=[1.0, 1.0, 1.0, 1.0, 1.0, 1.0, 1.0, 1.0, 1.0, 1.0, 1.0, 1.0, 1.0, 1.0, 1.0, 1.0, 1.0, 1.0, 1.0, 1.0, 1.0, 1.0, 1.0, 1.0, 1.0, 1.0, 1.0, 1.0, 1.0, 1.0, 1.0, 1.0, 1.0, 1.0, 1.0, 1.0, 1.0, 1.0, 1.0, 1.0, 1.0, 1.0, 1.0, 1.0, 1.0, 1.0, 1.0, 1.0, 1.0, 1.0, 1.0, 1.0, 1.0, 1.0, 1.0, 1.0, 1.0, 1.0, 1.0, 1.0, 1.0, 1.0, 1.0, 1.0, 1.0, 1.0, 1.0, 1.0, 1.0, 1.0, 1.0, 1.0, 1.0, 1.0, 1.0, 1.0, 1.0, 1.0, 1.0, 1.0, 1.0, 1.0, 1.0, 1.0, 1.0, 1.0, 1.0, 1.0, 1.0, 1.0, 1.0, 1.0, 1.0, 1.0, 1.0, 1.0, 1.0, 1.0, 1.0, 1.0, 1.0, 1.0, 1.0, 1.0, 1.0, 1.0, 1.0, 1.0, 1.0, 1.0, 1.0, 1.0, 1.0, 1.0, 1.0, 1.0, 1.0, 1.0, 1.0, 1.0, 1.0, 1.0, 1.0, 1.0, 1.0, 1.0, 1.0, 1.0, 1.0, 1.0, 1.0, 1.0, 1.0, 1.0, 1.0, 1.0, 1.0, 1.0, 1.0, 1.0, 1.0, 1.0, 1.0, 1.0, 1.0, 1.0, 1.0, 1.0, 1.0, 1.0, 1.0, 1.0, 1.0, 1.0, 1.0, 1.0, 1.0, 1.0, 1.0, 1.0, 1.0, 1.0, 1.0, 1.0, 1.0, 1.0, 1.0, 1.0, 1.0, 1.0, 1.0, 1.0, 1.0, 1.0, 1.0, 1.0, 1.0, 1.0, 1.0, 1.0, 1.0, 1.0, 1.0, 1.0, 1.0, 1.0, 1.0, 1.0, 1.0, 1.0, 1.0, 1.0, 1.0, 1.0, 1.0, 1.0, 1.0, 1.0, 1.0, 1.0, 1.0, 1.0, 1.0, 1.0, 1.0, 1.0, 1.0, 1.0, 1.0, 1.0, 1.0, 1.0, 1.0, 1.0, 1.0, 1.0, 1.0, 1.0, 1.0, 1.0, 1.0, 1.0, 1.0, 1.0, 1.0, 1.0, 1.0, 1.0, 1.0, 1.0, 1.0, 1.0, 1.0, 1.0, 1.0, 1.0, 1.0, 1.0, 1.0, 1.0, 1.0, 1.0, 1.0, 1.0, 1.0, 1.0, 1.0, 1.0, 1.0, 1.0, 1.0, 1.0, 1.0, 1.0, 1.0, 1.0, 1.0, 1.0, 1.0, 1.0, 1.0, 1.0, 1.0, 1.0, 1.0, 1.0, 1.0, 1.0, 1.0, 1.0, 1.0, 1.0, 1.0, 1.0, 1.0, 1.0, 1.0], "Y"=array[280 elements]}]
  in  "dead time":dbl=3.7e-08
  out "Optical Depth":cluster{"Y":dbl[], "Y":dbl[]}[](graph) caption="XY Graph"
  out "RingBuffer offline far":dbl[][](array[numeric])
  out "RingBuffer aerosol far":dbl[][](array[numeric])
  in  "Weather":T3(tab)=enum."Pulse Energy (Micro Joule)"
  in  "Temperature (C)":dbl=15.0
  out "Temperature (C)":dbl(graph)=15.0
  in  "Pressure (mbar or hPa)":dbl=832.0
  out "Pressure (mb)":dbl(graph)=832.0
  out "Relative Humdity (%)":dbl(graph)=40.0
  out "Pulse Energy (Micro Joule)":T4(graph)={"Online Pulse Energy"=3.281811428571428, "Pulse Energy Offline"=3.294908571428571}
  out "?":cluster{"mean":dbl, "mean":dbl}(graph)={"mean"=51080.0, "mean"=0.0}
  out "Index":i32=65
  out "Aerosol Smoothed":dbl[](array[numeric])=[25567.789655172426, 462.14482758620676, 690.513793103448, 902.9862068965513, 1074.1034482758619, 1191.9620689655176, 1254.3103448275865, 1254.1379310344828, 1211.8068965517243, 1150.593103448276, 1069.610344827586, 986.7827586206894, 916.5827586206894, 851.2758620689651, 784.4620689655169, 729.1103448275858, 683.3413793103445, 634.1965517241376, 570.8482758620687, 487.21379310344815, 406.7931034482758, 358.49310344827586, 343.2965517241379, 333.3965517241379, 312.93793103448274, 281.6, 245.02758620689664, 213.13793103448285, 183.544827586207, 156.23448275862074, 134.56206896551728, 117.81724137931037, 105.55517241379312, 94.00344827586207, 83.97241379310346, 75.0, 68.42758620689654, 63.71379310344825, 57.23448275862067, 54.65862068965515, 54.11724137931033, 52.26896551724136, 50.893103448275845, 49.07931034482757, 43.779310344827564, 35.56896551724137, 29.196551724137922, 23.848275862068963, 18.475862068965522, 17.97586206896552, 17.182758620689654, 14.927586206896555, 15.441379310344832, 15.234482758620697, 14.213793103448284, 13.375862068965525, 13.61379310344828, 12.017241379310349, 9.648275862068969, 9.406896551724142, 8.058620689655175, 8.258620689655174, 9.244827586206899, 7.362068965517245, 8.57586206896552, 9.082758620689658, 5.63448275862069, 5.589655172413794, 6.468965517241382, 6.375862068965519, 5.182758620689656, 4.365517241379312, 6.117241379310347, 4.824137931034484, 4.851724137931034, 4.768965517241378, 2.63448275862069, 4.096551724137932, 4.662068965517241, 2.4413793103448276, 2.4931034482758623, 4.279310344827587, 3.948275862068966, 2.675862068965518, 2.33448275862069, 2.7586206896551735, 3.8000000000000016, 4.158620689655174, 4.220689655172414, 4.67586206896552, 4.196551724137933, 3.1241379310344835, 1.862068965517242, 2.782758620689656, 3.041379310344828, 2.3931034482758626, 1.8137931034482766, 2.010344827586208, 3.7241379310344844, 3.5310344827586215, 1.7275862068965522, 0.5758620689655178, 1.4862068965517248, 3.2862068965517257, 2.9000000000000012, -0.013793103448275335, -0.5379310344827579, 1.4137931034482767, 1.5586206896551733, 0.0068965517241386665, 0.26551724137931104, 1.555172413793104, 1.6310344827586214, 2.131034482758621, 1.6793103448275866, 0.24137931034482818, 1.3137931034482762, 1.5137931034482761, 0.3517241379310351, -0.31379310344827566, -0.1310344827586205, 0.3344827586206903, -0.14482758620689587, 0.3000000000000006, 1.1931034482758627, 0.8000000000000006, -0.1999999999999994, 0.8793103448275866, 1.7137931034482763, -1.3931034482758629, -0.5896551724137937, 1.0482758620689663, -0.1517241379310339, 0.6310344827586213, 0.0206896551724145, 0.8068965517241388, 1.9551724137931041, 1.1103448275862076, 0.13103448275862128, -0.3896551724137925, 0.8965517241379317, 1.5896551724137937, 1.1827586206896559, 1.2965517241379316, 0.2793103448275868, -0.337931034482758, -0.33448275862068905, -1.1896551724137925, -0.8241379310344822, 0.16206896551724198, 0.7896551724137937, -0.06896551724137878, -0.38965517241379255, -0.5448275862068956, -0.31379310344827493, -0.09310344827586148, -0.4103448275862063, 1.1793103448275868, 1.7758620689655178, 0.9793103448275868, -0.7344827586206889, -0.3931034482758613, 1.3310344827586214, -0.4586206896551712, -1.3586206896551714, -0.02413793103448217, -1.0172413793103445, -0.8172413793103446, 0.5827586206896558, -0.2551724137931029, -0.637931034482758, -0.07931034482758563, -0.24827586206896493, 0.5965517241379317, 1.3000000000000007, 0.7517241379310351, 0.8241379310344834, 0.8034482758620696, 0.9793103448275867, 1.6172413793103455, 2.0103448275862075, 1.6517241379310348, 0.3827586206896557, 0.12413793103448337, 0.6137931034482764, 0.6448275862068972, 0.5379310344827593, 0.23448275862069023, 1.0482758620689665, 0.3931034482758632, 0.2896551724137938, 1.1344827586206903, 0.07586206896551781, 0.5482758620689661, -1.0482758620689654, -0.586206896551724, 1.5172413793103456, 0.8793103448275867, 1.3103448275862075, -0.15517241379310276, 0.5034482758620696, 0.6413793103448282, -0.2241379310344822, 0.7586206896551729, -0.08275862068965459, 0.4172413793103454, -0.43793103448275794, -0.39999999999999925, -0.16551724137930968, -1.1068965517241374, -1.2689655172413785, -1.210344827586206, 0.3310344827586213, 1.4689655172413802, 1.6482758620689666, -0.027586206896551224, -0.6034482758620685, -1.0724137931034476, -1.3551724137931027, 0.148275862068966, -0.5896551724137926, -0.9896551724137924, -0.2999999999999993, 0.875862068965518, 1.048275862068966, -0.03793103448275803, -0.01034482758620631, -0.9310344827586197, -1.0517241379310334, -0.19655172413793046, 0.4068965517241385, 0.11034482758620734, -1.8827586206896547, -0.5620689655172406, 0.22413793103448354, -0.9758620689655166, 0.05862068965517303, 0.13793103448275923, -1.0068965517241373, -0.7172413793103443, 0.42758620689655236, 0.555172413793104, -0.2689655172413787, -1.5689655172413786, -0.9310344827586201, -0.8517241379310339, 0.46896551724138, 0.6137931034482768, -1.9517241379310337, -1.2551724137931028, 0.8551724137931037, 0.5862068965517244, -1.037931034482758, -0.7896551724137925, 0.2724137931034488, -0.9310344827586206, -1.5034482758620689, -0.6517241379310339, -0.6068965517241374, -0.9862068965517233, -1.5103448275862057, -2.472413793103448, -0.7551724137931037, 1.3758620689655177, -0.23103448275862026, 0.020689655172414168, 0.027586206896552223, 0.17586206896551748, 0.10344827586206917, -1.1724137931034477, -1.33103448275862, -0.434482758620689, 0.6344827586206903, 0.07586206896551784, 0.4862068965517247, 1.6724137931034488, 1.2344827586206903]
  out "Off-Line  Bin Readings":dbl[](array[numeric])=[51252.0, 640.0, 895.0, 1057.0, 1242.0, 1414.0, 1541.0, 1545.0, 1503.0, 1370.0, 1349.0, 1265.0, 1226.0, 1190.0, 1075.0, 1069.0, 961.0, 997.0, 912.0, 770.0, 719.0, 611.0, 603.0, 595.0, 572.0, 521.0, 500.0, 445.0, 417.0, 399.0, 392.0, 415.0, 375.0, 373.0, 333.0, 350.0, 343.0, 338.0, 317.0, 313.0, 302.0, 298.0, 293.0, 299.0, 309.0, 290.0, 275.0, 285.0, 259.0, 270.0, 283.0, 284.0, 268.0, 256.0, 273.0, 258.0, 240.0, 294.0, 265.0, 260.0, 286.0, 240.0, 284.0, 257.0, 236.0, 306.0, 261.0, 288.0, 261.0, 284.0, 234.0, 295.0, 229.0, 241.0, 258.0, 271.0, 260.0, 245.0, 245.0, 248.0, 225.0, 263.0, 268.0, 256.0, 247.0, 247.0, 257.0, 258.0, 259.0, 275.0, 268.0, 271.0, 255.0, 269.0, 270.0, 273.0, 247.0, 236.0, 279.0, 272.0, 257.0, 270.0, 274.0, 252.0, 272.0, 261.0, 238.0, 240.0, 251.0, 253.0, 237.0, 251.0, 257.0, 256.0, 271.0, 241.0, 251.0, 264.0, 245.0, 239.0, 273.0, 232.0, 256.0, 243.0, 236.0, 266.0, 257.0, 262.0, 230.0, 261.0, 263.0, 272.0, 262.0, 256.0, 273.0, 248.0, 283.0, 273.0, 269.0, 271.0, 240.0, 253.0, 244.0, 245.0, 259.0, 249.0, 269.0, 247.0, 227.0, 259.0, 241.0, 240.0, 251.0, 287.0, 236.0, 259.0, 255.0, 267.0, 241.0, 268.0, 241.0, 284.0, 270.0, 260.0, 245.0, 275.0, 273.0, 227.0, 239.0, 273.0, 257.0, 237.0, 261.0, 237.0, 235.0, 226.0, 272.0, 256.0, 222.0, 250.0, 272.0, 263.0, 254.0, 261.0, 248.0, 281.0, 257.0, 271.0, 255.0, 271.0, 276.0, 240.0, 251.0, 230.0, 255.0, 227.0, 262.0, 239.0, 259.0, 278.0, 245.0, 267.0, 265.0, 229.0, 246.0, 233.0, 254.0, 259.0, 277.0, 219.0, 251.0, 251.0, 230.0, 243.0, 243.0, 279.0, 248.0, 266.0, 256.0, 261.0, 271.0, 257.0, 257.0, 259.0, 256.0, 251.0, 245.0, 209.0, 275.0, 242.0, 250.0, 255.0, 244.0, 252.0, 246.0, 250.0, 234.0, 245.0, 255.0, 239.0, 241.0, 259.0, 258.0, 246.0, 268.0, 253.0, 275.0, 266.0, 231.0, 256.0, 253.0, 258.0, 229.0, 256.0, 278.0, 258.0, 228.0, 238.0, 241.0, 246.0, 232.0, 222.0, 253.0, 225.0, 272.0, 250.0, 259.0, 259.0, 233.0, 248.0, 249.0, 277.0, 251.0, 255.0, 246.0, 269.0, 279.0, 245.0, 235.0]
  out "Off-Line Smoothed":dbl[](array[numeric])=[25538.924063116356, 471.08875739645, 706.0769230769237, 924.1124260355036, 1093.9280078895467, 1207.2524654832346, 1262.7159763313607, 1258.989151873767, 1212.514792899408, 1143.0207100591717, 1061.8096646942806, 978.7455621301783, 903.6094674556219, 834.1015779092709, 763.0285996055234, 694.127218934912, 630.3461538461545, 570.4260355029589, 506.73175542406307, 438.31262327416164, 378.10059171597635, 342.36686390532554, 328.7278106508876, 317.9753451676529, 301.3264299802761, 276.6410256410255, 246.88954635108462, 217.05226824457577, 188.9043392504929, 163.91124260355014, 142.31755424063107, 123.62327416173568, 107.27712031558187, 92.93491124260356, 81.9378698224852, 75.10453648915187, 69.9260355029586, 64.89644970414206, 60.924063116370846, 58.15187376725842, 56.466469428007926, 56.64595660749511, 67.43688362919134, 254.96646942800788, 547.010848126233, 589.5059171597634, 313.2287968441814, 65.35502958579883, 19.460552268244577, 17.158777120315573, 15.410256410256398, 13.949704142011825, 14.483234714003935, 13.692307692307683, 12.43688362919131, 12.927021696252456, 12.369822485207091, 10.179487179487172, 9.002958579881653, 9.087771203155812, 9.13017751479289, 8.027613412228794, 6.814595660749508, 6.331360946745562, 7.428994082840237, 7.414201183431954, 5.886587771203159, 6.1725838264299835, 5.877712031558188, 5.110453648915189, 4.276134122287971, 3.38856015779093, 3.917159763313612, 3.7159763313609497, 3.767258382643001, 3.2337278106508895, 2.226824457593691, 2.3303747534516805, 2.0739644970414224, 1.2396449704142016, 1.3481262327416181, 2.5167652859960574, 2.3017751479289963, 2.6094674556213038, 2.6863905325443804, 2.663708086785012, 2.8017751479289963, 2.7810650887573987, 3.0936883629191363, 2.5641025641025674, 2.1232741617357016, 1.360946745562131, 0.4930966469428018, 1.335305719921107, 1.9092702169625269, 1.694280078895464, 1.9506903353057203, 2.2080867850098636, 2.9644970414201204, 3.170611439842212, 2.281065088757399, 1.2120315581854053, 1.4930966469428015, 1.3925049309664703, 0.2761341222879693, -0.1883629191321489, 0.9704142011834335, 1.7899408284023677, 1.4497041420118348, 1.3520710059171606, 0.48915187376725977, 0.3037475345167665, 0.7169625246548333, 0.9289940828402371, 0.5197238658777122, -0.21499013806706024, 1.1883629191321525, 0.6992110453648939, -0.2406311637080864, -0.5917159763313606, -1.1844181459566068, -0.18244575936883528, -0.6745562130177507, -0.552268244575936, 0.7820512820512827, -0.2011834319526623, -1.5424063116370803, -0.42307692307692213, 0.0759368836291926, -0.782051282051281, 0.47140039447731885, 1.0591715976331373, -0.12721893491124187, -0.011834319526626363, 0.4230769230769239, 0.44181459566075054, 0.5108481262327429, 0.20315581854043507, -0.3925049309664685, -0.07692307692307607, -0.11932938856015715, -0.5019723865877707, -0.14694280078895383, 0.05818540433925145, -0.8392504930966463, -1.4280078895463502, -1.1163708086785, -1.397435897435897, -1.2909270216962516, -0.8875739644970402, -0.43293885601577786, -1.1429980276134108, -1.9329388560157776, -0.883629191321498, 0.5216962524654838, -0.03254437869822446, -0.5601577909270211, 0.5424063116370816, -0.06410256410256282, -1.6449704142011812, -1.6577909270216948, -0.802761341222879, 0.06213017751479394, -0.8944773175542389, -1.9467455621301757, -1.1321499013806695, -1.1400394477317548, -1.3836291913214986, -1.2771203155818538, -0.9201183431952659, -0.49605522682445663, -0.27120315581853943, -0.6558185404339242, -0.4112426035502949, -0.04240631163707986, -0.7465483234713997, -1.0591715976331355, -0.6942800788954626, 0.06410256410256523, 0.680473372781066, 0.43293885601577997, -0.10157790927021591, -0.6489151873767255, -0.5266272189349109, 0.016765285996056124, -0.5276134122287961, -0.7859960552268239, -0.14299802761341152, -0.4526627218934905, -0.928994082840236, -0.879684418145956, -0.6410256410256407, -0.6301775147928984, -0.7297830374753442, -0.8451676528599608, -0.10453648915187375, 0.31459566074950746, -0.5848126232741613, -0.02071005917159685, -0.2682445759368828, -0.5187376725838257, -0.4536489151873761, -0.48915187376725777, 0.40631163708086865, 0.04832347140039539, -0.2692307692307682, -0.43885601577909167, -0.1370808678500975, -0.18047337278106368, -0.8254437869822473, -0.5907297830374744, -0.29191321499013717, -0.8333333333333326, -1.0078895463510842, 0.014792899408284904, -0.8530571992110451, -1.7623274161735698, -1.634122287968441, -1.6222879684418137, -1.475345167652859, -1.9506903353057177, -2.418145956607492, -1.2662721893491107, -0.2386587771203144, -0.6232741617356988, -0.8530571992110441, -0.7830374753451664, -0.38165680473372693, -0.815581854043392, -1.19723865877712, -0.03648915187376672, -0.30867850098619226, -1.8047337278106488, -1.7199211045364877, -1.162721893491124, -1.2840236686390525, -0.7248520710059162, -0.09960552268244485, -0.8964497041420109, -1.1824457593688353, -0.5216962524654823, 0.16765285996055324, 0.2544378698224861, -0.7820512820512807, -0.6913214990138054, -0.9723865877712025, -0.8451676528599599, -0.010848126232740535, -0.6942800788954628, -1.057199211045364, -0.06311637080867771, 0.04635108481262362, -0.8382642998027605, -0.757396449704141, -0.7820512820512812, -1.5197238658777092, -1.9132149901380644, -1.2988165680473365, -0.5729783037475336, -0.5049309664694273, -0.9546351084812617, -0.9861932938856006, -0.5266272189349102, -0.2169625246548313, -0.34516765285995954, 0.08284023668639148, -0.3737672583826418, -0.10848126232741462, 0.2218934911242617, -0.782051282051281, -0.6005917159763303, 0.2583826429980287, 0.3313609467455631, 0.036489151873768125, 0.5187376725838274, 1.064102564102565, 0.8974358974358982]
  out "On-Line  Smoothed":dbl[](array[numeric])=[20165.23562992128, 335.83405511811026, 469.6037401574801, 575.6116141732278, 638.9482283464561, 666.4590551181095, 663.315354330708, 629.3429133858263, 576.093897637795, 517.8370078740155, 457.5466535433069, 401.2129921259843, 352.4570866141734, 308.6322834645672, 270.85177165354355, 236.83602362204752, 207.89704724409472, 182.70118110236237, 156.92165354330723, 129.95019685039378, 106.74940944881891, 91.97480314960627, 83.94429133858264, 79.25728346456688, 72.90492125984247, 63.32618110236215, 53.78681102362199, 45.05846456692909, 37.76122047244091, 31.828149606299196, 26.33503937007874, 22.759251968503946, 20.016141732283476, 16.702165354330724, 15.281889763779544, 14.228740157480328, 12.209055118110246, 11.153937007874026, 10.251377952755917, 9.78484251968505, 9.37440944881891, 9.290748031496076, 10.335039370078754, 21.00039370078739, 37.835039370078675, 36.902952755905446, 17.198228346456673, 4.5131889763779505, 4.192322834645665, 3.245472440944882, 2.3468503937007874, 2.245472440944882, 1.7484251968503952, 2.054527559055118, 2.223818897637794, 2.1775590551181088, 1.8557086614173226, 0.6716535433070878, 0.8458661417322855, 1.740551181102364, 1.2385826771653559, 0.7956692913385843, 0.6598425196850403, 1.2513779527559066, 1.6775590551181119, 1.6450787401574818, 1.3557086614173235, 0.7769685039370082, 1.0092519685039378, 2.2169291338582666, 2.3478346456692907, 1.9049212598425194, 1.8232283464566919, 1.4147637795275605, 1.027952755905514, 0.29271653543307224, 0.147047244094489, 0.43346456692913515, 0.6775590551181108, 0.3783464566929135, 0.2297244094488201, -0.441535433070864, -0.3066929133858251, 0.6588582677165361, 0.4364173228346466, 1.1746062992125983, 0.9875984251968501, 0.5161417322834664, 0.930511811023624, 0.10767716535433203, -0.23877952755905402, -0.28011811023621946, 0.1588582677165366, 0.12933070866141894, 0.30846456692913504, 0.6706692913385831, -0.2112204724409436, -0.40413385826771486, -0.6187007874015733, -0.2761811023622035, -0.3145669291338574, 0.16574803149606365, 0.46594488188976446, -0.5921259842519672, -0.5911417322834633, -0.35492125984251865, 0.38622047244094515, 1.0082677165354337, 0.12244094488189178, -0.9661417322834627, -0.7712598425196838, 0.43149606299212756, 0.865551181102364, 0.5348425196850406, -0.2181102362204717, -0.9838582677165346, -0.3076771653543294, 0.17755905511811176, -0.5025590551181087, -0.5812992125984233, -0.6905511811023607, -0.7102362204724402, -0.24763779527559, 0.04468503937007948, 0.057480314960631294, 0.07125984251968667, 0.1529527559055127, -0.693503937007873, -0.6885826771653533, 0.07519685039370172, 0.022047244094489594, 0.32224409448819097, 0.02303149606299376, -1.2358267716535443, -1.2860236220472454, -0.28799212598425106, 0.08110236220472568, 0.04370078740157587, -0.9366141732283461, -0.9917322834645662, -0.04291338582677058, 0.23267716535433175, 0.2956692913385837, -0.022244094488188218, 0.18740157480315023, 0.12736220472441023, -0.4799212598425185, -0.3529527559055107, 0.3094488188976389, 0.6381889763779538, 0.08897637795275687, 0.2651574803149621, 0.43248031496063133, 0.3596456692913401, 0.19429133858267872, -0.39724409448818815, -0.49370078740157397, 0.1401574803149616, -0.14035433070865988, -0.4572834645669276, 0.026968503937009308, 0.24842519685039544, 0.3645669291338596, 0.23956692913385902, 0.8350393700787404, 0.8507874015748037, 0.8655511811023638, 0.6509842519685054, -0.14625984251968419, -0.040944881889762835, 0.6647637795275604, 0.1706692913385841, 0.05059055118110378, 0.8970472440944901, 0.26220472440945053, -0.16496062992125887, -0.41988188976377866, -0.9602362204724397, -0.816535433070865, -0.3155511811023614, -0.06850393700787308, 0.07322834645669452, 0.0171259842519699, -0.044881889763778465, 0.6214566929133871, 0.894094488188978, 0.9275590551181115, 0.5240157480314969, -0.22795275590551098, -0.5783464566929121, -0.8992125984251946, -0.6728346456692897, -0.7062992125984238, -0.34114173228346273, -0.9248031496063005, -1.0320866141732299, -0.02322834645669203, -0.10098425196850307, 0.984645669291339, 0.35472440944881967, -0.8883858267716521, -0.18661417322834536, 0.36456692913385924, 0.4196850393700797, -0.35885826771653384, -0.43464566929133697, -0.06751968503936928, -0.16496062992125904, -0.09901574803149521, 0.08996062992126097, 0.24645669291338693, -0.00944881889763692, 0.12440944881889852, -0.09015748031495954, -0.7584645669291319, -0.4120078740157459, 0.5259842519685047, 0.902952755905513, 0.5751968503937028, 0.025000000000001354, 0.31633858267716686, 0.7444881889763802, 0.08700787401574978, -0.3234251968503927, -0.15413385826771583, -0.18759842519684922, -0.5350393700787386, -0.5586614173228336, 0.017125984251969373, -0.17578740157480235, -0.005511811023621083, -0.12755905511810917, -0.038976377952754826, 0.260236220472442, -0.2692913385826764, -0.018307086614172435, 0.12637795275590624, 0.150984251968505, -0.3007874015748019, -0.5045275590551173, 0.29665354330708743, 0.7425196850393716, 0.48366141732283613, 0.16968503937007895, 0.07519685039370104, 0.01712598425196977, -0.22696850393700682, 0.005314960629922594, -0.37952755905511704, -0.002559055118109499, 1.066338582677166, 0.6125984251968513, -0.8096456692913372, -0.7712598425196838, -0.4031496062992109, -0.8372047244094474, -0.7112204724409437, -0.08720472440944738, 0.022047244094489438, 0.36259842519685187, 0.6027559055118122, -0.5360236220472431, -0.33228346456692776, -0.32736220472440763, -0.09704724409448656, 0.6834645669291343, 0.6568897637795279, 0.14311023622047353, -0.36870078740157364, -0.5576771653543298, 0.45905511811023614, 1.1293307086614175, 1.2297244094488202, 0.018110236220473253, -0.8657480314960622, -0.3529527559055098, -0.6836614173228326]
  out "On-Line Bin Readings":dbl[](array[numeric])=[42763.0, 637.0, 919.0, 1087.0, 1221.0, 1369.0, 1339.0, 1288.0, 1251.0, 1146.0, 1037.0, 957.0, 909.0, 830.0, 740.0, 674.0, 663.0, 563.0, 526.0, 489.0, 380.0, 362.0, 375.0, 364.0, 346.0, 304.0, 311.0, 270.0, 262.0, 245.0, 236.0, 254.0, 299.0, 247.0, 226.0, 193.0, 258.0, 214.0, 231.0, 223.0, 231.0, 219.0, 219.0, 204.0, 215.0, 213.0, 203.0, 218.0, 217.0, 198.0, 208.0, 240.0, 195.0, 217.0, 220.0, 213.0, 208.0, 222.0, 199.0, 210.0, 229.0, 205.0, 207.0, 203.0, 197.0, 198.0, 239.0, 204.0, 198.0, 205.0, 206.0, 221.0, 201.0, 229.0, 224.0, 215.0, 206.0, 210.0, 217.0, 212.0, 208.0, 215.0, 203.0, 216.0, 208.0, 200.0, 223.0, 191.0, 206.0, 213.0, 200.0, 223.0, 233.0, 215.0, 212.0, 213.0, 184.0, 194.0, 230.0, 241.0, 203.0, 236.0, 190.0, 206.0, 228.0, 190.0, 205.0, 213.0, 186.0, 220.0, 172.0, 190.0, 214.0, 216.0, 211.0, 223.0, 202.0, 204.0, 247.0, 210.0, 219.0, 215.0, 193.0, 206.0, 212.0, 207.0, 197.0, 205.0, 226.0, 189.0, 204.0, 234.0, 221.0, 194.0, 192.0, 201.0, 205.0, 236.0, 197.0, 222.0, 204.0, 209.0, 211.0, 222.0, 210.0, 217.0, 225.0, 212.0, 183.0, 213.0, 191.0, 214.0, 213.0, 211.0, 234.0, 208.0, 205.0, 218.0, 189.0, 193.0, 191.0, 195.0, 209.0, 218.0, 218.0, 192.0, 209.0, 220.0, 220.0, 218.0, 228.0, 215.0, 221.0, 215.0, 240.0, 209.0, 231.0, 217.0, 207.0, 223.0, 205.0, 230.0, 236.0, 240.0, 210.0, 233.0, 204.0, 196.0, 242.0, 202.0, 197.0, 213.0, 188.0, 216.0, 216.0, 218.0, 219.0, 231.0, 204.0, 193.0, 225.0, 200.0, 178.0, 209.0, 212.0, 194.0, 222.0, 215.0, 205.0, 211.0, 243.0, 222.0, 209.0, 231.0, 195.0, 235.0, 196.0, 225.0, 209.0, 212.0, 207.0, 211.0, 233.0, 229.0, 198.0, 204.0, 183.0, 224.0, 182.0, 203.0, 205.0, 207.0, 195.0, 183.0, 204.0, 185.0, 212.0, 199.0, 191.0, 205.0, 190.0, 209.0, 231.0, 223.0, 199.0, 193.0, 204.0, 223.0, 187.0, 219.0, 216.0, 182.0, 205.0, 205.0, 232.0, 233.0, 209.0, 187.0, 231.0, 201.0, 178.0, 194.0, 218.0, 207.0, 242.0, 189.0, 217.0, 224.0, 224.0, 204.0, 229.0, 221.0, 198.0, 232.0, 231.0, 236.0, 212.0, 206.0, 189.0]
  out "Range Corrected Altitude Array":dbl[](array[numeric])=[5625.0, 22500.0, 50625.0, 90000.0, 140625.0, 202500.0, 275625.0, 360000.0, 455625.0, 562500.0, 680625.0, 810000.0, 950625.0, 1102500.0, 1265625.0, 1440000.0, 1625625.0, 1822500.0, 2030625.0, 2250000.0, 2480625.0, 2722500.0, 2975625.0, 3240000.0, 3515625.0, 3802500.0, 4100625.0, 4410000.0, 4730625.0, 5062500.0, 5405625.0, 5760000.0, 6125625.0, 6502500.0, 6890625.0, 7290000.0, 7700625.0, 8122500.0, 8555625.0, 9000000.0, 9455625.0, 9922500.0, 10400625.0, 10890000.0, 11390625.0, 11902500.0, 12425625.0, 12960000.0, 13505625.0, 14062500.0, 14630625.0, 15210000.0, 15800625.0, 16402500.0, 17015625.0, 17640000.0, 18275625.0, 18922500.0, 19580625.0, 20250000.0, 20930625.0, 21622500.0, 22325625.0, 23040000.0, 23765625.0, 24502500.0, 25250625.0, 26010000.0, 26780625.0, 27562500.0, 28355625.0, 29160000.0, 29975625.0, 30802500.0, 31640625.0, 32490000.0, 33350625.0, 34222500.0, 35105625.0, 36000000.0, 36905625.0, 37822500.0, 38750625.0, 39690000.0, 40640625.0, 41602500.0, 42575625.0, 43560000.0, 44555625.0, 45562500.0, 46580625.0, 47610000.0, 48650625.0, 49702500.0, 50765625.0, 51840000.0, 52925625.0, 54022500.0, 55130625.0, 56250000.0, 57380625.0, 58522500.0, 59675625.0, 60840000.0, 62015625.0, 63202500.0, 64400625.0, 65610000.0, 66830625.0, 68062500.0, 69305625.0, 70560000.0, 71825625.0, 73102500.0, 74390625.0, 75690000.0, 77000625.0, 78322500.0, 79655625.0, 81000000.0, 82355625.0, 83722500.0, 85100625.0, 86490000.0, 87890625.0, 89302500.0, 90725625.0, 92160000.0, 93605625.0, 95062500.0, 96530625.0, 98010000.0, 99500625.0, 101002500.0, 102515625.0, 104040000.0, 105575625.0, 107122500.0, 108680625.0, 110250000.0, 111830625.0, 113422500.0, 115025625.0, 116640000.0, 118265625.0, 119902500.0, 121550625.0, 123210000.0, 124880625.0, 126562500.0, 128255625.0, 129960000.0, 131675625.0, 133402500.0, 135140625.0, 136890000.0, 138650625.0, 140422500.0, 142205625.0, 144000000.0, 145805625.0, 147622500.0, 149450625.0, 151290000.0, 153140625.0, 155002500.0, 156875625.0, 158760000.0, 160655625.0, 162562500.0, 164480625.0, 166410000.0, 168350625.0, 170302500.0, 172265625.0, 174240000.0, 176225625.0, 178222500.0, 180230625.0, 182250000.0, 184280625.0, 186322500.0, 188375625.0, 190440000.0, 192515625.0, 194602500.0, 196700625.0, 198810000.0, 200930625.0, 203062500.0, 205205625.0, 207360000.0, 209525625.0, 211702500.0, 213890625.0, 216090000.0, 218300625.0, 220522500.0, 222755625.0, 225000000.0, 227255625.0, 229522500.0, 231800625.0, 234090000.0, 236390625.0, 238702500.0, 241025625.0, 243360000.0, 245705625.0, 248062500.0, 250430625.0, 252810000.0, 255200625.0, 257602500.0, 260015625.0, 262440000.0, 264875625.0, 267322500.0, 269780625.0, 272250000.0, 274730625.0, 277222500.0, 279725625.0, 282240000.0, 284765625.0, 287302500.0, 289850625.0, 292410000.0, 294980625.0, 297562500.0, 300155625.0, 302760000.0, 305375625.0, 308002500.0, 310640625.0, 313290000.0, 315950625.0, 318622500.0, 321305625.0, 324000000.0, 326705625.0, 329422500.0, 332150625.0, 334890000.0, 337640625.0, 340402500.0, 343175625.0, 345960000.0, 348755625.0, 351562500.0, 354380625.0, 357210000.0, 360050625.0, 362902500.0, 365765625.0, 368640000.0, 371525625.0, 374422500.0, 377330625.0, 380250000.0, 383180625.0, 386122500.0, 389075625.0, 392040000.0, 395015625.0, 398002500.0, 401000625.0, 404010000.0, 407030625.0, 410062500.0, 413105625.0, 416160000.0, 419225625.0, 422302500.0, 425390625.0, 428490000.0, 431600625.0, 434722500.0, 437855625.0, 441000000.0]
  out "Altitude Array (km)":dbl[](array[numeric])=[0.075, 0.15, 0.22499999999999998, 0.3, 0.375, 0.45, 0.5249999999999999, 0.6, 0.6749999999999999, 0.7499999999999999, 0.825, 0.8999999999999999, 0.9749999999999999, 1.05, 1.125, 1.2, 1.275, 1.3499999999999999, 1.4249999999999998, 1.5, 1.575, 1.65, 1.7249999999999999, 1.7999999999999998, 1.8749999999999998, 1.95, 2.025, 2.1, 2.1750000000000003, 2.25, 2.325, 2.4, 2.475, 2.5500000000000003, 2.625, 2.7, 2.775, 2.85, 2.9250000000000003, 3.0, 3.075, 3.15, 3.225, 3.3000000000000003, 3.375, 3.45, 3.525, 3.6, 3.675, 3.75, 3.825, 3.9, 3.975, 4.05, 4.125, 4.2, 4.275, 4.35, 4.425, 4.5, 4.575, 4.65, 4.725, 4.8, 4.875, 4.95, 5.025, 5.1, 5.175, 5.25, 5.325, 5.4, 5.475, 5.55, 5.625, 5.7, 5.775, 5.85, 5.925, 6.0, 6.075, 6.15, 6.225, 6.3, 6.375, 6.45, 6.525, 6.6, 6.675, 6.75, 6.825, 6.9, 6.975, 7.05, 7.125, 7.2, 7.2749999999999995, 7.35, 7.425, 7.5, 7.575, 7.6499999999999995, 7.725, 7.8, 7.875, 7.95, 8.024999999999999, 8.1, 8.174999999999999, 8.249999999999998, 8.325, 8.399999999999999, 8.475, 8.549999999999999, 8.624999999999998, 8.7, 8.774999999999999, 8.85, 8.924999999999999, 8.999999999999998, 9.075, 9.149999999999999, 9.225, 9.299999999999999, 9.374999999999998, 9.45, 9.524999999999999, 9.6, 9.674999999999999, 9.749999999999998, 9.825, 9.899999999999999, 9.975, 10.049999999999999, 10.124999999999998, 10.2, 10.274999999999999, 10.35, 10.424999999999999, 10.499999999999998, 10.575, 10.649999999999999, 10.725, 10.799999999999999, 10.874999999999998, 10.95, 11.024999999999999, 11.1, 11.174999999999999, 11.249999999999998, 11.325, 11.399999999999999, 11.475, 11.549999999999999, 11.624999999999998, 11.7, 11.774999999999999, 11.85, 11.924999999999999, 11.999999999999998, 12.075, 12.149999999999999, 12.225, 12.299999999999999, 12.374999999999998, 12.45, 12.524999999999999, 12.6, 12.674999999999999, 12.749999999999998, 12.825, 12.899999999999999, 12.975, 13.049999999999999, 13.124999999999998, 13.2, 13.274999999999999, 13.35, 13.424999999999999, 13.499999999999998, 13.575, 13.649999999999999, 13.725, 13.799999999999999, 13.874999999999998, 13.95, 14.024999999999999, 14.1, 14.174999999999999, 14.249999999999998, 14.325, 14.399999999999999, 14.474999999999998, 14.549999999999999, 14.624999999999998, 14.7, 14.774999999999999, 14.849999999999998, 14.924999999999999, 14.999999999999998, 15.075, 15.149999999999999, 15.224999999999998, 15.299999999999999, 15.374999999999998, 15.45, 15.524999999999999, 15.599999999999998, 15.674999999999999, 15.749999999999998, 15.825, 15.899999999999999, 15.974999999999998, 16.05, 16.125, 16.2, 16.275, 16.349999999999998, 16.424999999999997, 16.5, 16.575, 16.65, 16.724999999999998, 16.799999999999997, 16.875, 16.95, 17.025, 17.099999999999998, 17.174999999999997, 17.25, 17.325, 17.4, 17.474999999999998, 17.549999999999997, 17.625, 17.7, 17.775, 17.849999999999998, 17.924999999999997, 18.0, 18.075, 18.15, 18.224999999999998, 18.299999999999997, 18.375, 18.45, 18.525, 18.599999999999998, 18.674999999999997, 18.75, 18.825, 18.9, 18.974999999999998, 19.049999999999997, 19.125, 19.2, 19.275, 19.349999999999998, 19.424999999999997, 19.5, 19.575, 19.65, 19.724999999999998, 19.799999999999997, 19.875, 19.95, 20.025, 20.099999999999998, 20.174999999999997, 20.25, 20.325, 20.4, 20.474999999999998, 20.549999999999997, 20.625, 20.7, 20.775, 20.849999999999998, 20.924999999999997, 21.0]
  out "Offline Pulse Energy":dbl=3.283532857142857
  out "Online Pulse Energy":dbl=3.281811428571428
  in  "Instrument Control":T5(tab)=enum."Wavemeter"
  in  "ILX Address On":dbl=1.0 min=0.0 step=1.0
  in  "ILX Address Off":dbl=2.0 min=0.0 step=1.0
  in  "OnLineLD":dbl=169.7
  in  "OffLineLD":dbl=172.62
  in  "Pulse B Polarity":enum32{"Low", "High"}(ring)=enum."High"
  in  "Pulse A Delay(ns)":u32=1040 min=80 max=327600
  in  "Pulse B Delay(ns)":u32=170000 min=80 max=327600 step=1
  in  "Accumulation Delay(ns)":u32=10 min=10 max=1270 step=1
  in  "Sync Pulse Polarity":enum32{"Low", "High"}(ring)=enum."High"
  in  "Pulse A Polarity":enum32{"Low", "High"}(ring)=enum."High"
  in  "Number of Bins":u32=280 min=2 max=4095 step=1
  in  "Number of Accumulates":u32=10000 min=1 max=32767 step=1
  in  "Time Resolution Per Bin(ns)":u32=500 min=5 max=1063 step=1
  in  "Lambda On Set (nm)":dbl=828.198 format="%.5f"
  out "Lambda On Read (nm)":dbl=828.1979407398044 format="%.5f"
  out "Lambda Off Read (nm)":dbl=828.2039208197817 format="%.5f"
  in  "Lambda Off Set (nm)":dbl=828.29765 format="%#.5f"
  in  "Bristol In":i32=5
  out "Bristol Out":i32=1221
  out "AB_DIF":dbl=-5.926019559865381e-05 format="%#_15g"
  out "NONAB_DIF":dbl=-0.09372918021824717 format="%#_15g"
  out "Wavelength Lock Online":bool=TRUE
  out "Wavelength Lock Offline":bool=TRUE
  in  "calculate absorption cross sections":bool
  in  "Smoothing Range":dbl=150.0
  in  "Total DIAL Integration Time (Minutes)":i32=3
  in  "Data Reads (number of loops)":i32=1
  in  "Total Aerosol Integration Time (Minutes)":dbl=0.5
  in  "Scalar Wait Time":u32=500
  out "Smoothed Bins":dbl=2.0
  in  "NewportIn":string
  in  "logging":bool
  out "Newport Device Key":string="1918-R 15120"
  in  "SampleSize":i32=2
  out "NewportRef":refnum<k24>
  in  "Switch Comm Port":refnum<visa-resource-name>="COM3"
  out "FF_On_Ref":refnum<file>
  out "FF_On_Ptr":i64=1091376 format="%.2p"
  out "FF_Off_Ref":refnum<file>
  out "FF_Off_Ptr":i64=1091376 format="%.2p"
  out "NF_On_Ref":refnum<file>
  out "NF_On_Ptr":i64=1091376 format="%.2p"
  out "NF_Off_Ref":refnum<file>
  out "NF_Off_Ptr":i64=1091376 format="%.2p"
  out "DataOpen":bool=TRUE
  out "File Path_Far Field (out)":string="C:\\Users\\H2ODial\\Desktop\\SharedTeleWVData\\160812FF\\19"
  out "File Path_Near Field (out)":string="C:\\Users\\H2ODial\\Desktop\\SharedTeleWVData\\160812NF\\19"
  in  "Data File DIR (in)":string="C:\\Users\\H2ODial\\Desktop\\SharedTeleWVData\\"
  in  "bins":u32=280 min=2 max=4095 step=1
  out "y offset":u32=10
  in  "ns scale":u32=500
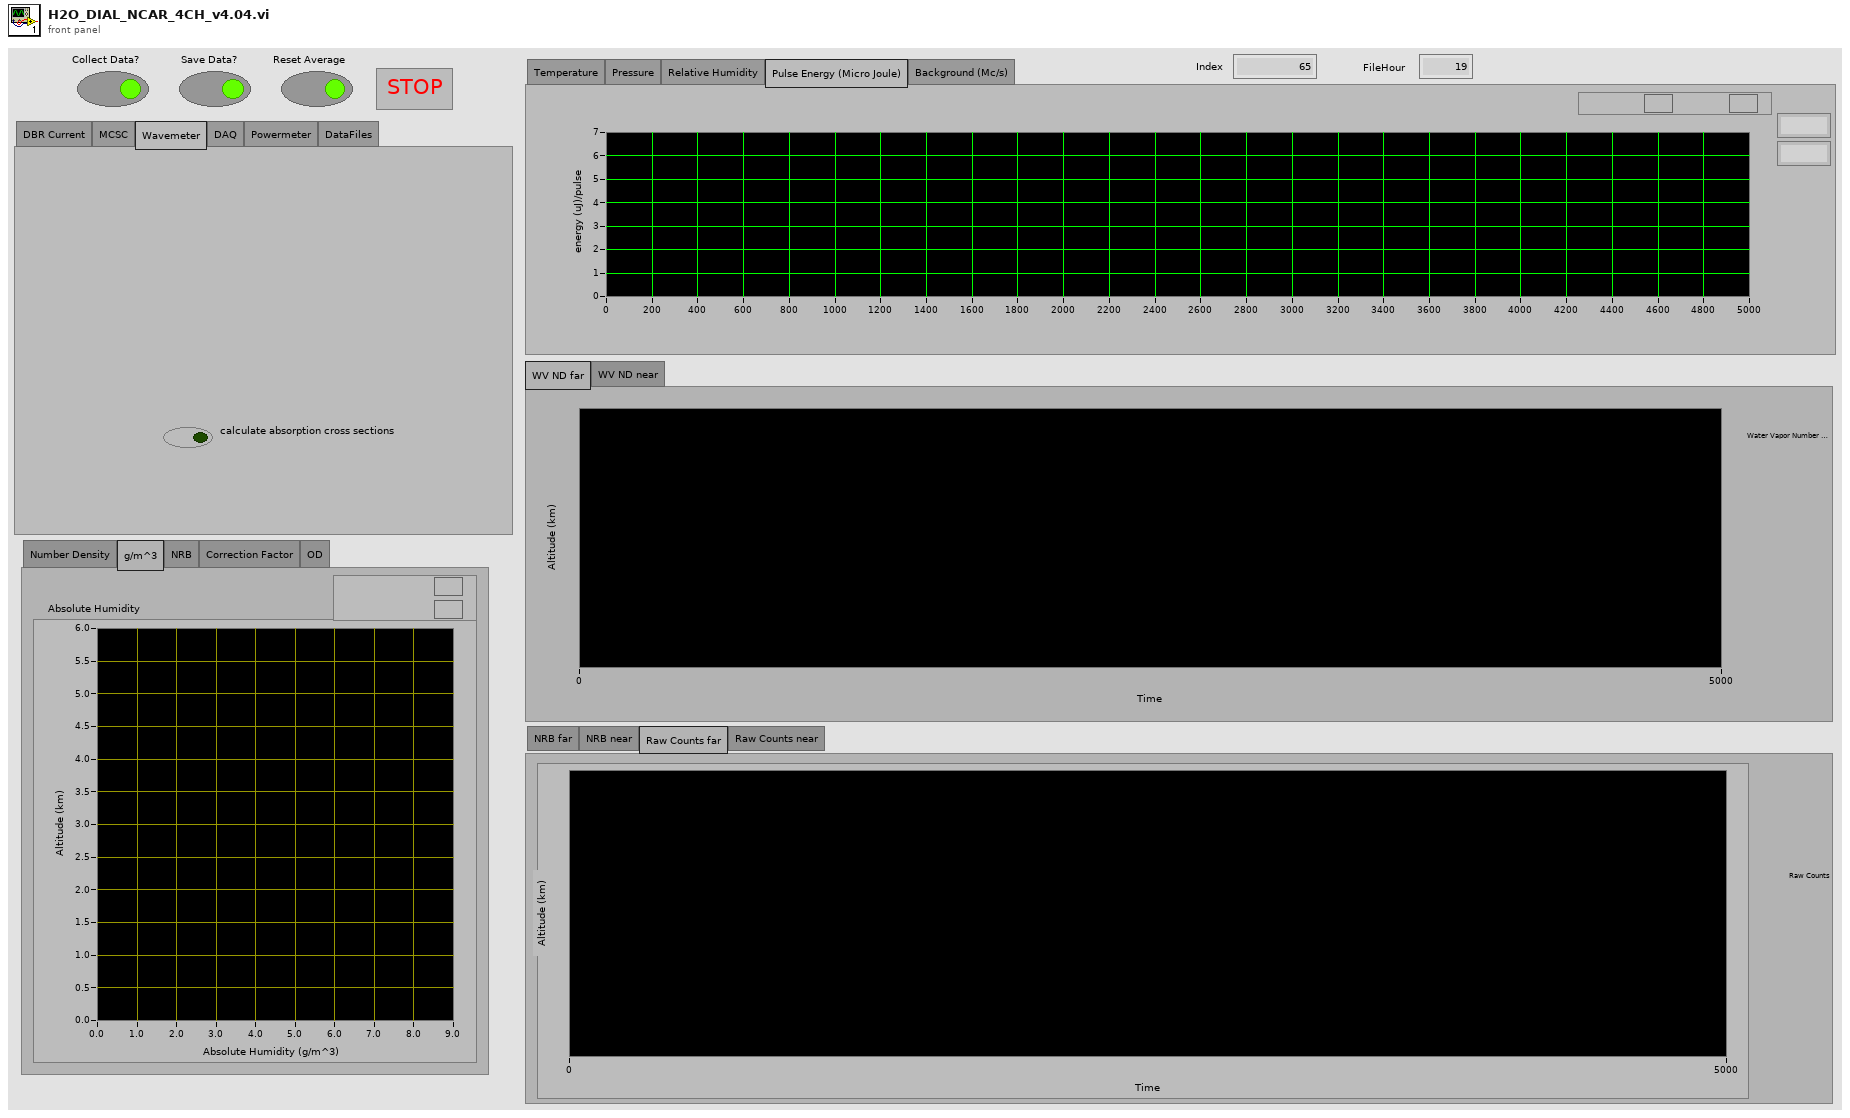
[diagram p1: front panel]
types:
  T1 = enum32{"NRB far", "NRB near", "Raw Counts far", "Raw Counts near"}
  T2 = enum32{"Number Density", "g/m^3", "NRB", "Correction Factor", "OD"}
  T3 = enum32{"Temperature", "Pressure", "Relative Humidity", "Pulse Energy (Micro Joule)", "Background (Mc/s)"}
  T4 = cluster{"Online Pulse Energy":dbl, "Pulse Energy Offline":dbl}
  T5 = enum32{"DBR Current", "MCSC", "Wavemeter", "DAQ", "Powermeter", "DataFiles"}
  T6 = enum16{"Initialize ILX", "Set ON T", "Set Off T", "Set ON I", "Set Off I", "Set On Lim", "Set Off Lim", "Read ILX", "TEC ON/OFF", "LASER ON/OFF", "Status?", "ILX OFF"}
  T7 = enum16{"open", "replace", "create", "open or create", "replace or create", "replace or create with confirmation"}
  T8 = typedef "LVDateTimeRec.ctl" = cluster{"fractional second":dbl, "second":i32, "minute":i32, "hour":i32, "day of month":i32, "month":i32, "year":i32, "day of week":i32, "day of year":i32, "DST":i32}
  T9 = cluster{"Online Pulse Energy":dbl, "Offline Pulse Energy":dbl}
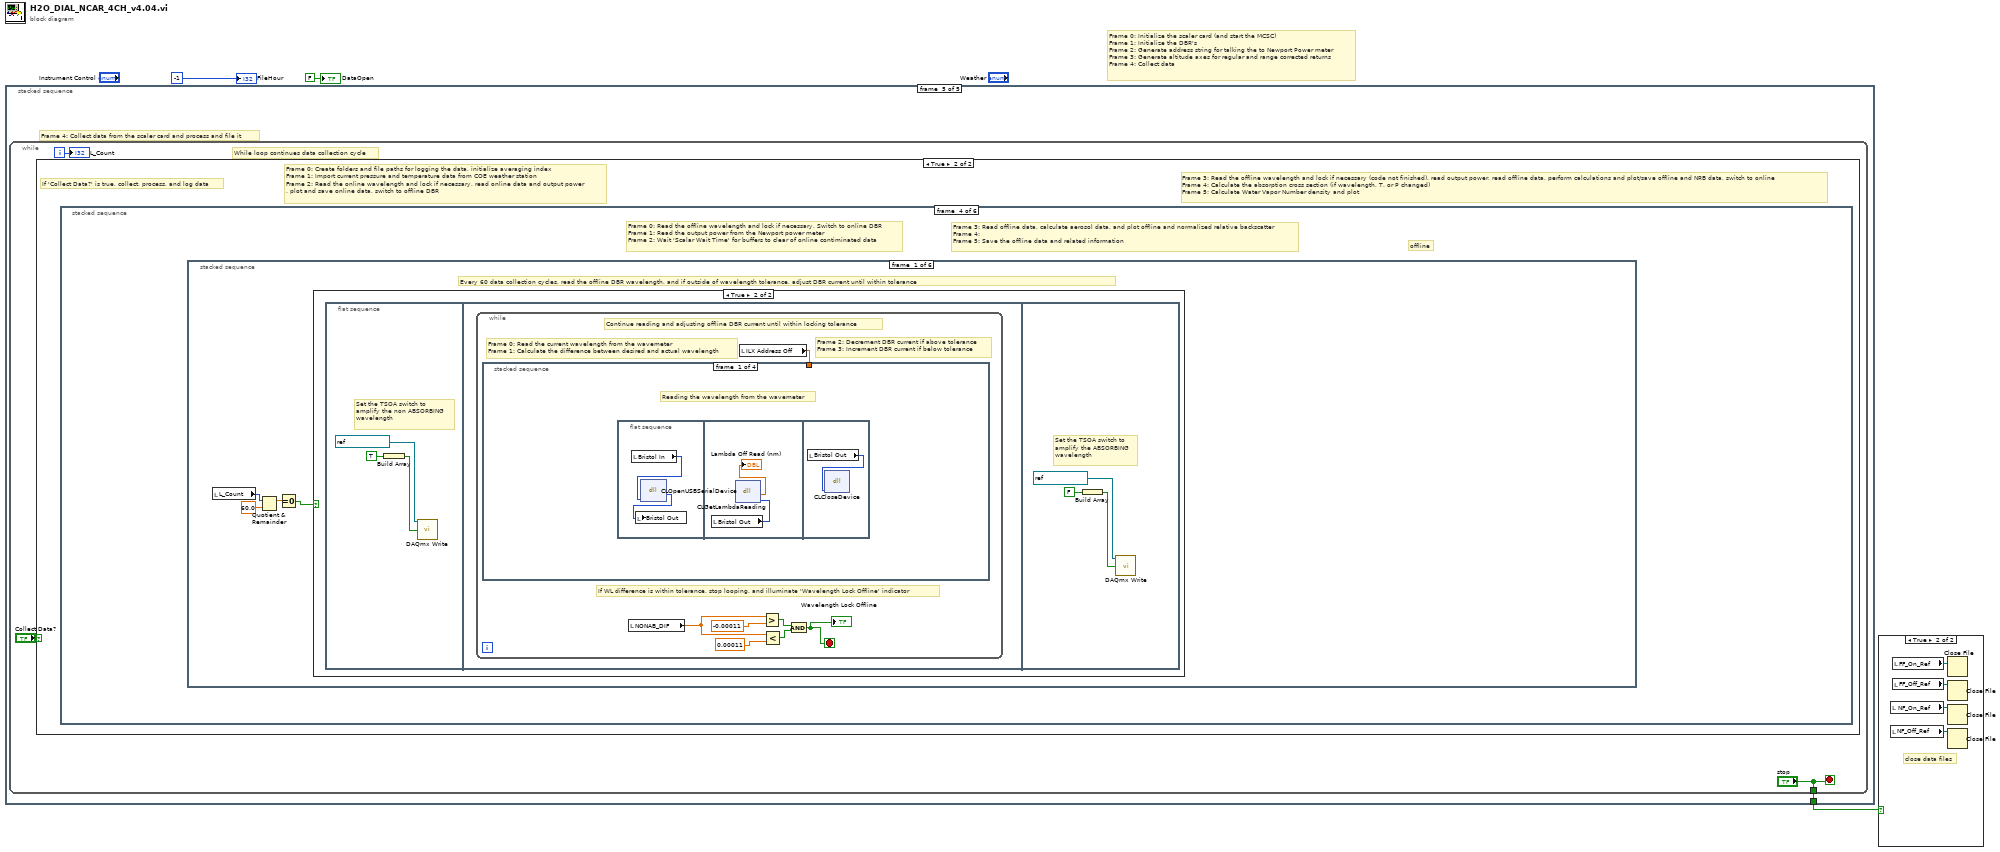
[diagram p0: block diagram]
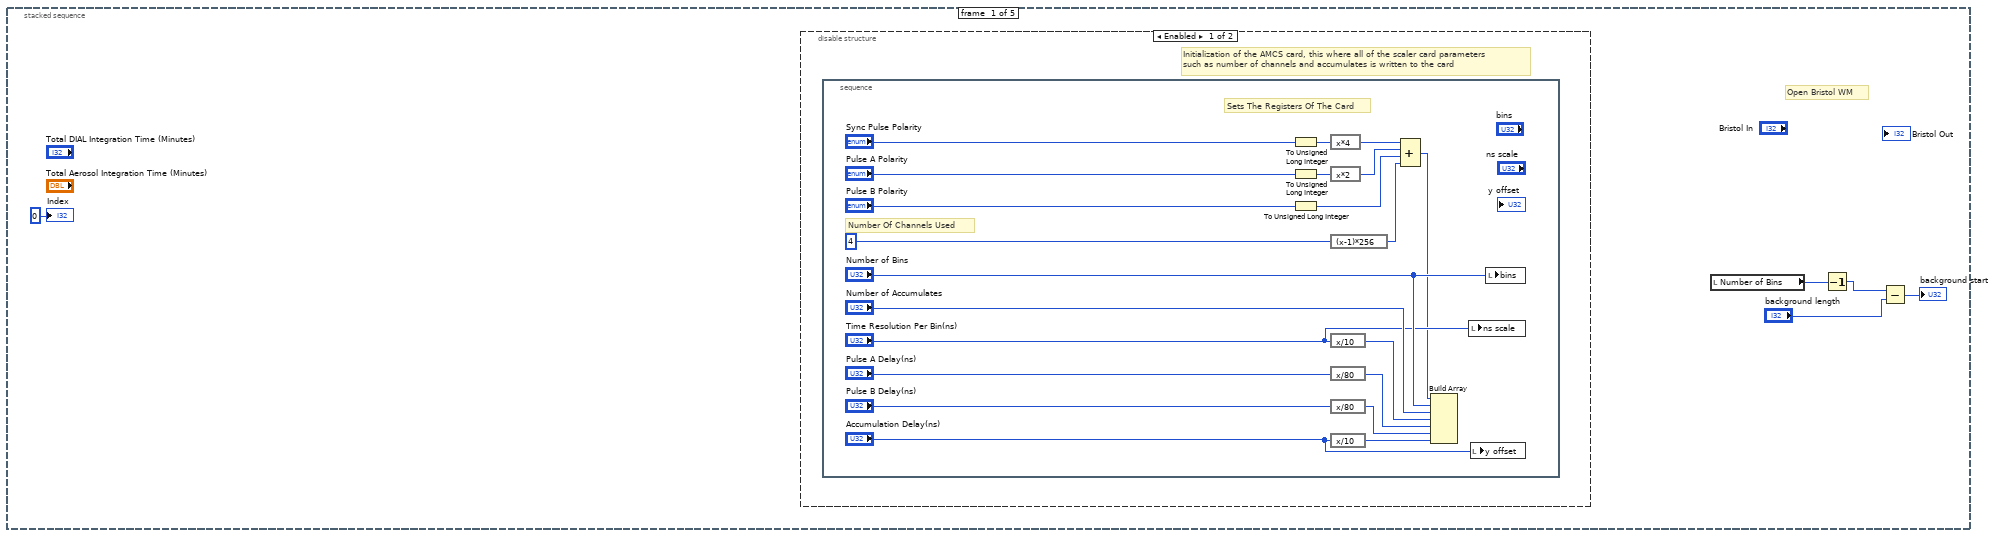
[diagram p3: hidden frame]
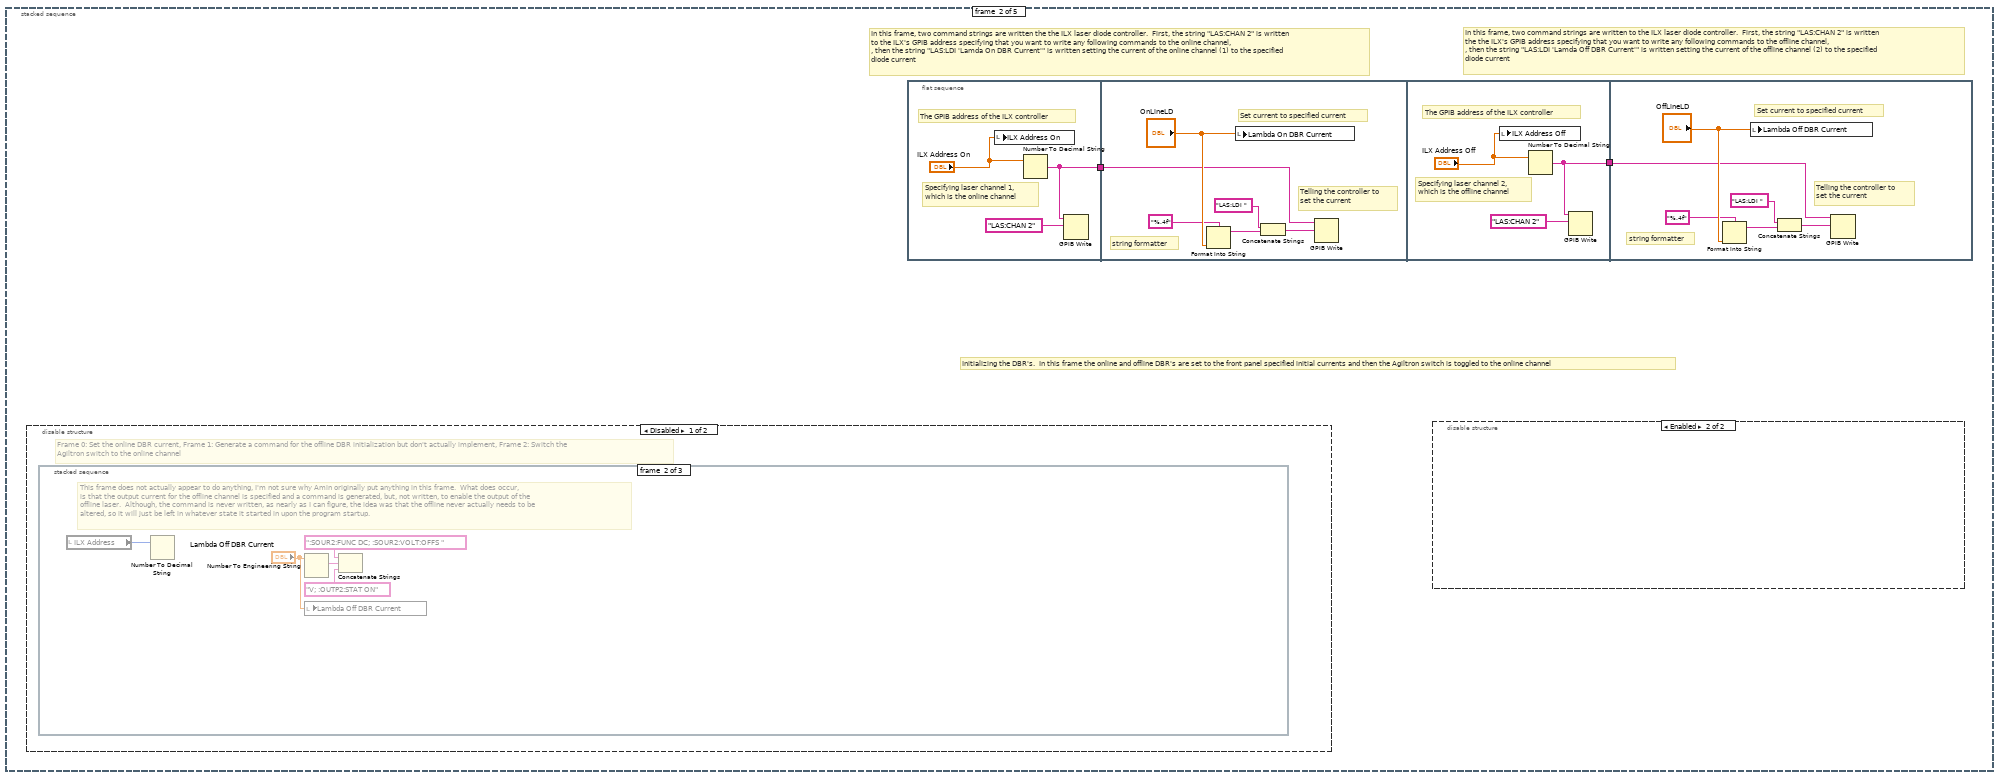
[diagram p5: hidden frame]
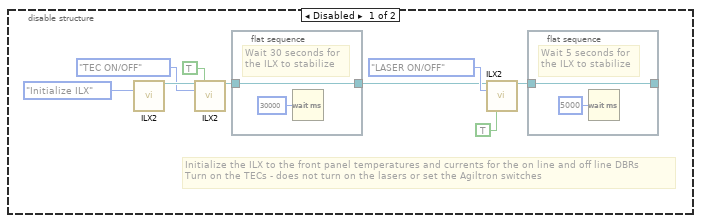
[diagram p6: hidden frame]
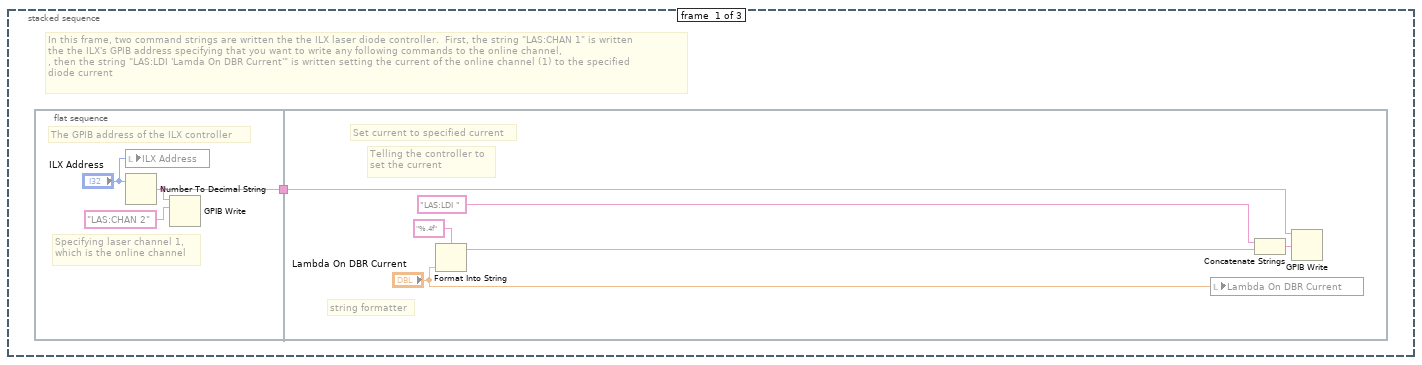
[diagram p7: hidden frame]
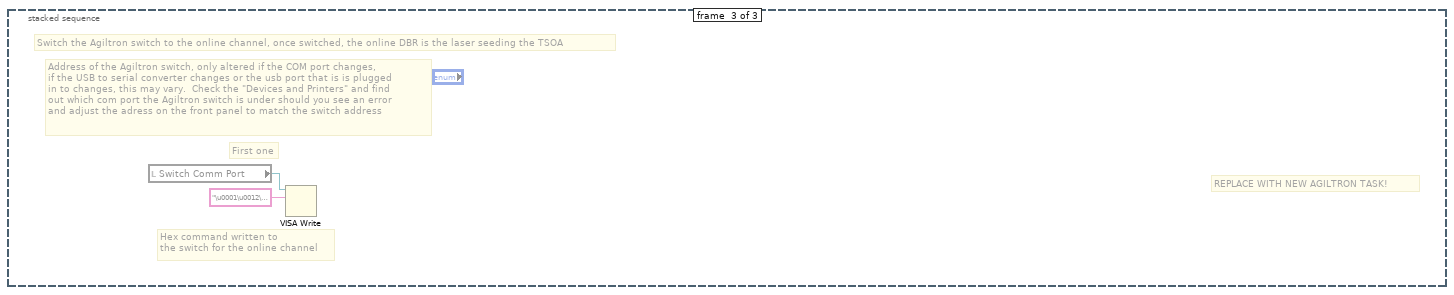
[diagram p8: hidden frame]
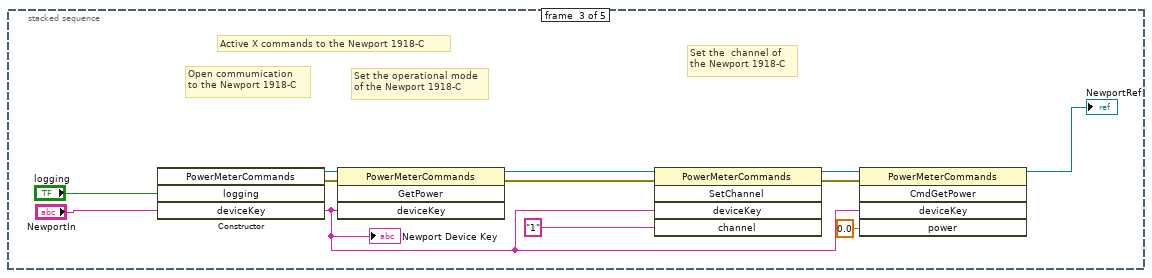
[diagram p10: hidden frame]
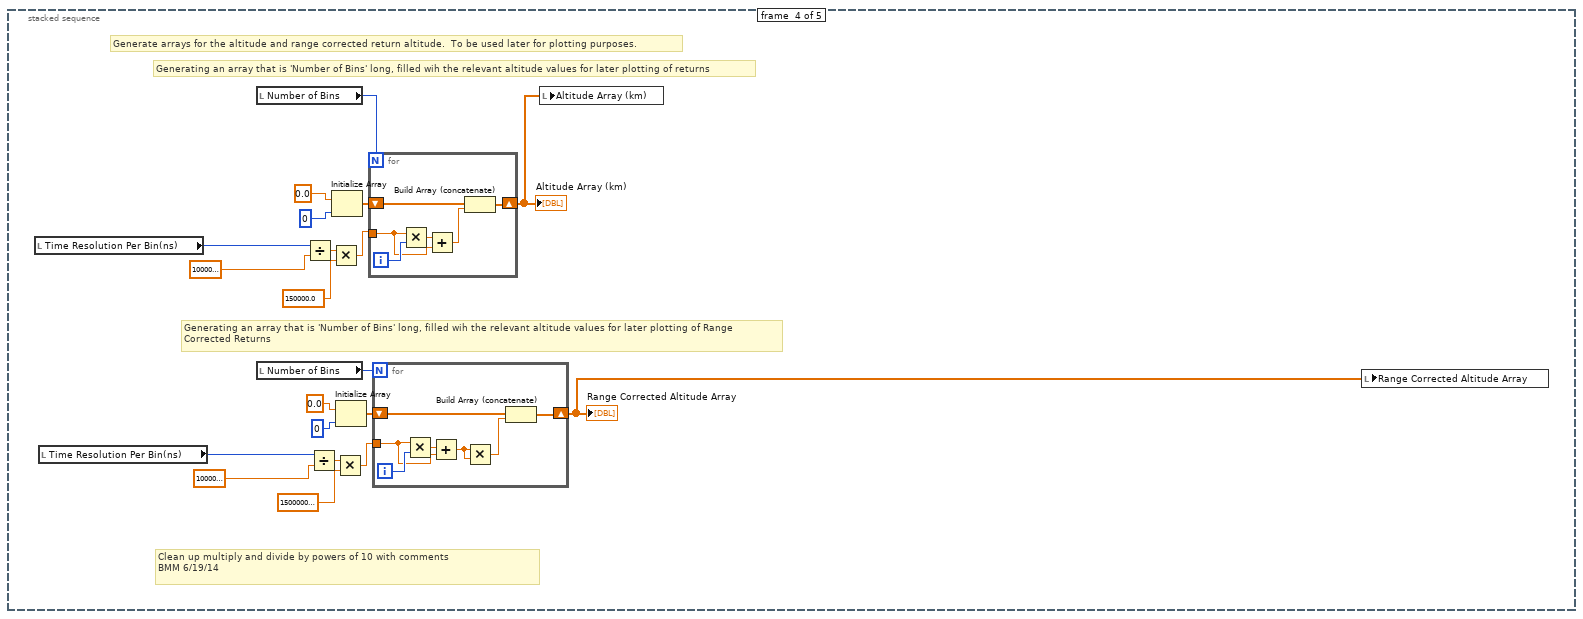
[diagram p11: hidden frame]
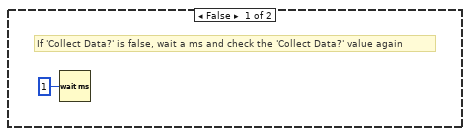
[diagram p12: hidden frame]
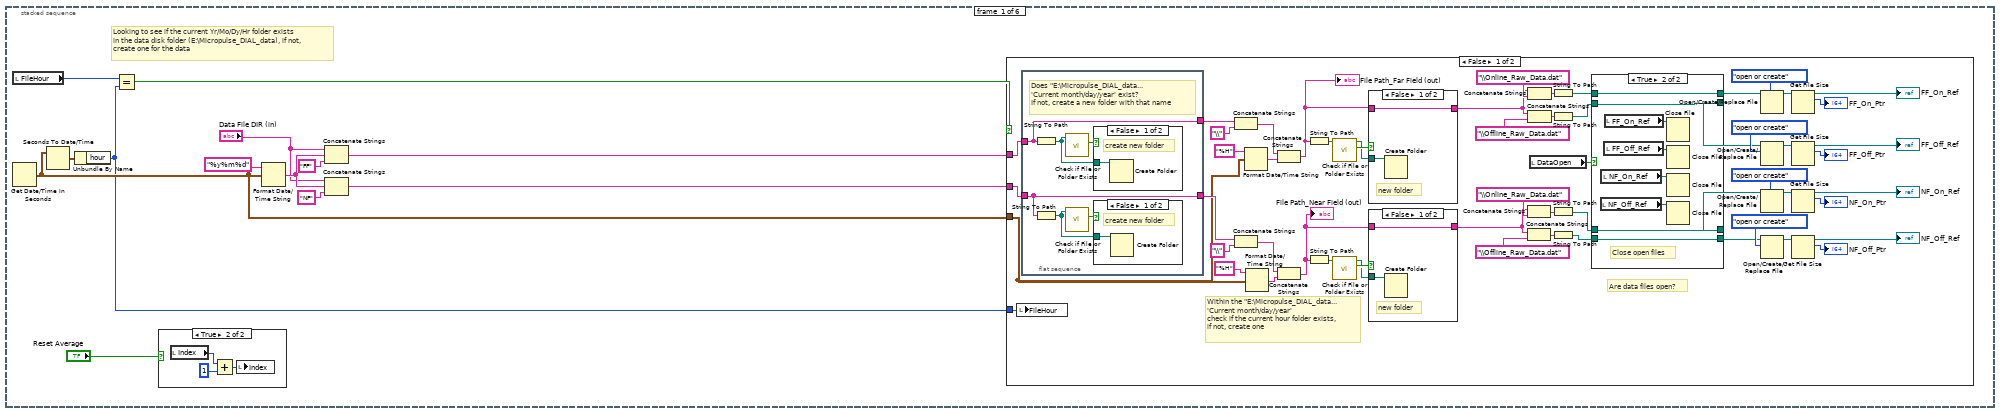
[diagram p13: hidden frame]
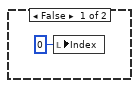
[diagram p20: hidden frame]
diagram:
  # "Frame 0: Initialize the scaler card (and start the MCSC)\nFrame 1: Initialize the DBR's\nFrame 2: Generate address string for talking the to Newport Power meter\nFrame 3: Generate altitude axes for regular and range corrected returns\nFrame 4: Collect data"
  n1 = stacked-sequence {
    tunnel: [_ _ _ _ w125] -> w3
    frame #0 {
      # "Open Bristol WM"
      n2 = disable-structure shown="Enabled" {
        frame Enabled {
          # "Initialization of the AMCS card, this where all of the scaler card parameters\nsuch as number of channels and accumulates is written to the card"
          n3 = stacked-sequence {
            frame #0 {
              # "Sets The Registers Of The Card"
              # "Number Of Channels Used"
              n4 = To Unsigned Long Integer(number="Sync Pulse Polarity") -> (unsigned 32bit integer=w9:u32)
              n5 = To Unsigned Long Integer(number="Pulse A Polarity") -> (unsigned 32bit integer=w13:u32)
              n6 = To Unsigned Long Integer(number="Pulse B Polarity") -> (unsigned 32bit integer=w11:u32)
              n7 = expression code="x*4"(w9) -> (w18:u32)
              n8 = expression code="x*2"(w13) -> (w17:u32)
              n9 = expression code="(x-1)*256"(u32 4 ("Number of Channels Used")) -> (w16:u32)
              n10 = expression code="x/10"("Time Resolution Per Bin(ns)") -> (w20:u32)
              n11 = expression code="x/80"("Pulse A Delay(ns)") -> (w27:u32)
              n12 = expression code="x/80"("Pulse B Delay(ns)") -> (w29:u32)
              n13 = expression code="x/10"("Accumulation Delay(ns)") -> (w28:u32)
              n14 = Compound Arithmetic op=ADD(w18, w17, w11, w16) -> (w15:u32)
              n15 = Build Array(w15, "Number of Bins", "Number of Accumulates", w20, w27, w29, w28) -> ()  [unwired: 1 out]
              n16 = local write "ns scale"("Time Resolution Per Bin(ns)") -> ()
              n17 = local write "y offset"("Accumulation Delay(ns)") -> ()
              n18 = local write "bins"("Number of Bins") -> ()
            }
          }
        }
        frame Disabled {
        }
      }
      n19 = local read "Number of Bins"() -> (w7:u32)
      n20 = Decrement(x=w7) -> (x-1=w6:u32)
      n21 = Subtract(x=w6, y="background length") -> (x-y=→"background start":u32)
      "Index" <- 0 ("Index")
    }
    frame #1 {
      # "In this frame, two command strings are written to the ILX laser diode controller.  First, the string \"LAS:CHAN 2\" is written\nthe the ILX's GPIB address specifying that you want to write any following commands to the offline channel,\n, then the string \"LAS:LDI 'Lamda Off DBR Current'\" is written setting the current of the offline channel (2) to the specified \ndiode current"
      # "In this frame, two command strings are written the the ILX laser diode controller.  First, the string \"LAS:CHAN 2\" is written\nto the ILX's GPIB address specifying that you want to write any following commands to the online channel,\n, then the string \"LAS:LDI 'Lamda On DBR Current'\" is written setting the current of the online channel (1) to the specified \ndiode current"
      # "Initializing the DBR's.  In this frame the online and offline DBR's are set to the front panel specified initial currents and then the Agiltron switch is toggled to the online channel"
      n22 = disable-structure shown="Disabled" {
        frame Disabled {
          # "Frame 0: Set the online DBR current, Frame 1: Generate a command for the offline DBR initialization but don't actually implement, Frame 2: Switch the \nAgiltron switch to the online channel"
          n23 = stacked-sequence {
            frame #0 {
              # "In this frame, two command strings are written the the ILX laser diode controller.  First, the string \"LAS:CHAN 1\" is written\nthe the ILX's GPIB address specifying that you want to write any following commands to the online channel,\n, then the string \"LAS:LDI 'Lamda On DBR Current'\" is written setting the current of the online channel (1) to the specified \ndiode current"
              n24 = flat-sequence {
                tunnel: [w65] -> w63
                tunnel: w63 -> [w67]
                frame #0 {
                  # "The GPIB address of the ILX controller"
                  # "Specifying laser channel 1,\nwhich is the online channel"
                  n25 = local write "ILX Address"("ILX Address") -> ()
                  n26 = Number To Decimal String(number="ILX Address") -> (decimal integer string=w65:string)  [unwired: 1 in]
                  n27 = GPIB Write(0:w65, 1:"LAS:CHAN 2") -> ()  [unwired: 3 in, 2 out]
                }
                frame #1 {
                  # "Telling the controller to\nset the current"
                  # "string formatter"
                  # "Set current to specified current"
                  n28 = Format Into String(format string="%.4f" ("Format String"), "Lambda On DBR Current") -> (resulting string=w70:string)  [unwired: 2 in, 1 out]
                  n29 = local write "Lambda On DBR Current"("Lambda On DBR Current") -> ()
                  n30 = Concatenate Strings("LAS:LDI ", w70) -> (w71:string)
                  n31 = GPIB Write(0:w67, 1:w71) -> ()  [unwired: 3 in, 2 out]
                }
              }
            }
            frame #1 {
              # "This frame does not actually appear to do anything, I'm not sure why Amin originally put anything in this frame.  What does occur, \nis that the output current for the offline channel is specified and a command is generated, but, not written, to enable the output of the\noffline laser.  Although, the command is never written, as nearly as I can figure, the idea was that the offline never actually needs to be \naltered, so it will just be left in whatever state it started in upon the program startup."
              n32 = local read "ILX Address"() -> (w73:i32)
              n33 = Number To Decimal String(number=w73) -> ()  [unwired: 1 in, 1 out]
              n34 = Number To Engineering String(4:"Lambda Off DBR Current") -> (0:w77:string)  [unwired: 3 in]
              n35 = local write "Lambda Off DBR Current"("Lambda Off DBR Current") -> ()
              n36 = Concatenate Strings(":SOUR2:FUNC DC; :SOUR2:VOLT:OFFS ", w77, "V; :OUTP2:STAT ON") -> ()  [unwired: 1 out]
            }
            frame #2 {
              # "REPLACE WITH NEW AGILTRON TASK!"
              # "First one"
              # "Address of the Agiltron switch, only altered if the COM port changes,\nif the USB to serial converter changes or the usb port that is is plugged\nin to changes, this may vary.  Check the \"Devices and Printers\" and find \nout which com port the Agiltron switch is under should you see an error \nand adjust the adress on the front panel to match the switch address"
              # "Hex command written to \nthe switch for the online channel"
              # "Switch the Agiltron switch to the online channel, once switched, the online DBR is the laser seeding the TSOA"
              n37 = local read "Switch Comm Port"() -> (w78:refnum<visa-resource-name>)
              n38 = VISA Write(VISA resource name=w78, write buffer="\u0001\u0012\u0000\u0002") -> ()  [unwired: 1 in, 3 out]
            }
          }
        }
        frame Enabled {
        }
      }
      n39 = flat-sequence {
        tunnel: [w33] -> w31
        tunnel: w31 -> [w35]
        tunnel: [w41] -> w30
        tunnel: w30 -> [w44]
        frame #0 {
          # "The GPIB address of the ILX controller"
          # "Specifying laser channel 1,\nwhich is the online channel"
          n40 = local write "ILX Address On"("ILX Address On") -> ()
          n41 = Number To Decimal String(number="ILX Address On") -> (decimal integer string=w33:string)  [unwired: 1 in]
          n42 = GPIB Write(0:w33, 1:"LAS:CHAN 2") -> ()  [unwired: 3 in, 2 out]
        }
        frame #1 {
          # "Telling the controller to\nset the current"
          # "string formatter"
          # "Set current to specified current"
          n43 = Format Into String(format string="%.4f" ("Format String"), "OnLineLD") -> (resulting string=w38:string)  [unwired: 2 in, 1 out]
          n44 = local write "Lambda On DBR Current"("OnLineLD") -> ()
          n45 = Concatenate Strings("LAS:LDI ", w38) -> (w39:string)
          n46 = GPIB Write(0:w35, 1:w39) -> ()  [unwired: 3 in, 2 out]
        }
        frame #2 {
          # "The GPIB address of the ILX controller"
          # "Specifying laser channel 2,\nwhich is the offline channel"
          n47 = local write "ILX Address Off"("ILX Address Off") -> ()
          n48 = Number To Decimal String(number="ILX Address Off") -> (decimal integer string=w41:string)  [unwired: 1 in]
          n49 = GPIB Write(0:w41, 1:"LAS:CHAN 2") -> ()  [unwired: 3 in, 2 out]
        }
        frame #3 {
          # "Telling the controller to\nset the current"
          # "string formatter"
          # "Set current to specified current"
          n50 = Format Into String(format string="%.4f" ("Format String"), "OffLineLD") -> (resulting string=w47:string)  [unwired: 2 in, 1 out]
          n51 = local write "Lambda Off DBR Current"("OffLineLD") -> ()
          n52 = Concatenate Strings("LAS:LDI ", w47) -> (w48:string)
          n53 = GPIB Write(0:w44, 1:w48) -> ()  [unwired: 3 in, 2 out]
        }
      }
      n54 = disable-structure shown="Enabled" {
        frame Disabled {
          # "Initialize the ILX to the front panel temperatures and currents for the on line and off line DBRs\nTurn on the TECs - does not turn on the lasers or set the Agiltron switches"
          n55 = call "ILX2.vi"("ILX Command"=T6."Initialize ILX") -> ("Device Out"=w57:refnum<visa-resource-name>)  [unwired: 10 in, 4 out]
          n56 = call "ILX2.vi"("Device In"=w57, "TEC Control"=TRUE, "ILX Command"=T6."TEC ON/OFF") -> ("Device Out"=w54:refnum<visa-resource-name>)  [unwired: 8 in, 4 out]
          n57 = flat-sequence {
            tunnel: w54 -> [w61]
            tunnel: [w61] -> w51
            frame #0 {
              # "Wait 30 seconds for\nthe ILX to stabilize"
              n58 = Wait (ms)(milliseconds to wait=u32 30000) -> ()  [unwired: 1 out]
            }
          }
          n59 = call "ILX2.vi"("Device In"=w51, "ILX Command"=T6."LASER ON/OFF", "Laser Control"=TRUE ("TEC Control")) -> ("Device Out"=w50:refnum<visa-resource-name>)  [unwired: 8 in, 4 out]
          n60 = flat-sequence {
            tunnel: w50 -> [w59]
            tunnel: [w59] -> _
            frame #0 {
              # "Wait 5 seconds for\nthe ILX to stabilize"
              n61 = Wait (ms)(milliseconds to wait=u32 5000) -> ()  [unwired: 1 out]
            }
          }
        }
        frame Enabled {
        }
      }
    }
    frame #2 {
      # "Active X commands to the Newport 1918-C"
      # "Set the  channel of\nthe Newport 1918-C"
      # "Set the operational mode\nof the Newport 1918-C"
      # "Open commumication\nto the Newport 1918-C"
      n62 = constructor class="PowerMeterCommands"("logging"="logging", "deviceKey"="NewportIn") -> (reference out=w91:refnum<k24>, error out=w88:errorcluster, "deviceKey"=w83:string)  [unwired: 3 in, 2 out]
      "Newport Device Key" <- w83
      n63 = invoke class="PowerMeterCommands" method="GetPower"(reference=w91, error in=w88, "deviceKey"=w83) -> (reference out=w90:refnum<k24>, error out=w87:errorcluster)  [unwired: 1 in, 2 out]
      n64 = invoke class="PowerMeterCommands" method="SetChannel"(reference=w90, error in=w87, "deviceKey"=w83, "channel"="1") -> (reference out=w84:refnum<k24>, error out=w86:errorcluster)  [unwired: 1 in, 3 out]
      n65 = invoke class="PowerMeterCommands" method="CmdGetPower"(reference=w84, error in=w86, "deviceKey"=w83, "power"=sgl 0.0) -> (reference out=→"NewportRef":refnum<k24>)  [unwired: 1 in, 4 out]
    }
    frame #3 {
      # "Clean up multiply and divide by powers of 10 with comments\nBMM 6/19/14"
      # "Generating an array that is 'Number of Bins' long, filled wih the relevant altitude values for later plotting of Range \nCorrected Returns"
      # "Generating an array that is 'Number of Bins' long, filled wih the relevant altitude values for later plotting of returns"
      # "Generate arrays for the altitude and range corrected return altitude.  To be used later for plotting purposes."
      n66 = local read "Time Resolution Per Bin(ns)"() -> (w104:u32)
      n67 = local read "Time Resolution Per Bin(ns)"() -> (w94:u32)
      n68 = local read "Number of Bins"() -> (w107:u32)
      n69 = local read "Number of Bins"() -> (w97:u32)
      n70 = Divide(x=w104, y=1000000000.0) -> (x/y=w102:dbl)
      n71 = Divide(x=w94, y=1000000000.0) -> (x/y=w92:dbl)
      n72 = Multiply(x=w102, y=150000.0) -> (x*y=w105:dbl)
      n73 = Initialize Array(0.0, 0) -> (w110:dbl[])
      n74 = Multiply(x=w92, y=150000000.0) -> (x*y=w95:dbl)
      n75 = Initialize Array(0.0, 0) -> (w100:dbl[])
      n76 = for {
        N: w107 -> [_]
        shift-right: [w123] -> w108
        shift-left: w110 -> [w124]
        tunnel: w105 -> [w120]
        i -> [w122]
        n77 = Multiply(x=w120, y=w122) -> (x*y=w121:dbl)
        n78 = Add(x=w121, y=w120) -> (x+y=w119:dbl)
        n79 = Build Array (concatenate)(w124, w119) -> (w123:dbl[])
      }
      "Altitude Array (km)" <- w108
      n80 = for {
        N: w97 -> [_]
        shift-right: [w117] -> w98
        shift-left: w100 -> [w118]
        tunnel: w95 -> [w113]
        i -> [w116]
        n81 = Multiply(x=w113, y=w116) -> (x*y=w114:dbl)
        n82 = Add(x=w114, y=w113) -> (x+y=w112:dbl)
        n83 = Multiply(x=w112, y=w112) -> (x*y=w115:dbl)
        n84 = Build Array (concatenate)(w118, w115) -> (w117:dbl[])
      }
      "Range Corrected Altitude Array" <- w98
      n85 = local write "Altitude Array (km)"(w108) -> ()
      n86 = local write "Range Corrected Altitude Array"(w98) -> ()
    }
    frame #4 {
      # "Frame 4: Collect data from the scaler card and process and file it"
      n87 = while {
        tunnel: ["stop"] -> w125
        i -> [w126]
        stop <- "stop" stop-if-true
        # "While loop continues data collection cycle"
        n88 = case shown="True" "Collect Data?" {
          frame False {
            # "If 'Collect Data?' is false, wait a ms and check the 'Collect Data?' value again"
            n89 = Wait (ms)(milliseconds to wait=u32 1) -> ()  [unwired: 1 out]
          }
          frame True {
            # "Frame 3: Read the offline wavelength and lock if necessary (code not finished), read output power, read offline data, perform calculations and plot/save offline and NRB data, switch to online\nFrame 4: Calculate the absorption cross section (if wavelength, T, or P changed)\nFrame 5: Calculate Water Vapor Number density and plot"
            # "Frame 0: Create folders and file paths for logging the data, initialize averaging index\nFrame 1: Import current pressure and temperature data from COE weather station\nFrame 2: Read the online wavelength and lock if necessary, read online data and output power\n, plot and save online data, switch to offline DBR"
            # "If 'Collect Data?' is true, collect, process, and log data"
            n90 = stacked-sequence {
              frame #0 {
                # "Looking to see if the current Yr/Mo/Dy/Hr folder exists\nin the data disk folder (E:\\Micropulse_DIAL_data), if not,\ncreate one for the data"
                n91 = local read "FileHour"() -> (w139:i32)
                n92 = Get Date/Time In Seconds() -> (seconds since 1Jan1904=w131:timestamp)
                n93 = Seconds To Date/Time(time stamp (now)=w131) -> (date time rec=w141:T8)  [unwired: 1 in]
                n94 = Unbundle By Name(w141) -> ("hour"=w130:i32)
                n95 = Equal?(x=w139, y=w130) -> (x = y?=w140:bool)
                n96 = case shown="True" "Reset Average" {
                  frame False {
                    n97 = local write "Index"(0 ("Index")) -> ()
                  }
                  frame True {
                    n98 = local read "Index"() -> (w229:i32)
                    n99 = Add(x=w229, y=1) -> (x+y=w228:i32)
                    n100 = local write "Index"(w228) -> ()
                  }
                }
                n101 = Format Date/Time String(time format string (%c)="%y%m%d", seconds (now)=w131) -> (date/time string=w135:string)  [unwired: 1 in]
                n102 = Concatenate Strings("Data File DIR (in)", w135, "FF" ("string")) -> (w137:string)
                n103 = Concatenate Strings("Data File DIR (in)", w135, "NF" ("string")) -> (w132:string)
                n104 = case shown="False" w140 {
                  tunnel: w137 -> [w199 _]
                  tunnel: w132 -> [w198 _]
                  tunnel: w131 -> [w185 _]
                  tunnel: w130 -> [w161 _]
                  frame False {
                    # "Are data files open?"
                    # "Within the \"E:\\Micropulse_DIAL_data...\n'Current month/day/year' \ncheck if the current hour folder exists,\nif not, create one"
                    n105 = local write "FileHour"(w161) -> ()
                    n106 = flat-sequence {
                      tunnel: [w219] -> w186
                      tunnel: w199 -> [w218]
                      tunnel: w198 -> [w219]
                      tunnel: [w218] -> w187
                      frame #0 {
                        # "Does \"E:\\Micropulse_DIAL_data...\n'Current month/day/year' exist?\nIf not, create a new folder with that name"
                        n107 = String To Path(string=w218) -> (path=w223:path)
                        n108 = String To Path(string=w219) -> (path=w221:path)
                        n109 = call <vilib>:"Check if File or Folder Exists.vi"("path"=w223) -> ("file or folder exists?"=w222:bool)  [unwired: 8 in, 2 out]
                        n110 = call <vilib>:"Check if File or Folder Exists.vi"("path"=w221) -> ("file or folder exists?"=w220:bool)  [unwired: 8 in, 2 out]
                        n111 = case shown="False" w222 {
                          tunnel: w223 -> [w225 _]
                          frame False {
                            # "create new folder"
                            n112 = Create Folder(path (use dialog)=w225) -> ()  [unwired: 2 in, 3 out]
                          }
                          frame True {
                            # "Folder exists\ndo nothing"
                          }
                        }
                        n113 = case shown="False" w220 {
                          tunnel: w221 -> [w224 _]
                          frame False {
                            # "create new folder"
                            n114 = Create Folder(path (use dialog)=w224) -> ()  [unwired: 2 in, 3 out]
                          }
                          frame True {
                            # "Folder exists\ndo nothing"
                          }
                        }
                      }
                    }
                    n115 = Concatenate Strings(w187, "\\" ("string")) -> (w194:string)
                    n116 = Concatenate Strings(w186, "\\" ("string")) -> (w189:string)
                    n117 = Format Date/Time String(time format string (%c)="%H", seconds (now)=w185) -> (date/time string=w197:string)  [unwired: 1 in]
                    n118 = Format Date/Time String(time format string (%c)="%H", seconds (now)=w185) -> (date/time string=w192:string)  [unwired: 1 in]
                    n119 = Concatenate Strings(w194, w197) -> (w157:string)
                    "File Path_Far Field (out)" <- w157
                    n120 = Concatenate Strings(w189, w192) -> (w158:string)
                    "File Path_Near Field (out)" <- w158
                    n121 = String To Path(string=w157) -> (path=w195:path)
                    n122 = String To Path(string=w158) -> (path=w190:path)
                    n123 = call <vilib>:"Check if File or Folder Exists.vi"("path"=w195) -> ("file or folder exists?"=w184:bool, "dup path"=w182:path)  [unwired: 8 in, 1 out]
                    n124 = call <vilib>:"Check if File or Folder Exists.vi"("path"=w190) -> ("file or folder exists?"=w183:bool, "dup path"=w181:path)  [unwired: 8 in, 1 out]
                    n125 = case shown="False" w184 {
                      tunnel: w182 -> [w216 _]
                      tunnel: w157 -> [w215 w217]
                      tunnel: [w215 w217] -> w155
                      frame False {
                        # "new folder"
                        n126 = Create Folder(path (use dialog)=w216) -> ()  [unwired: 2 in, 3 out]
                      }
                      frame True {
                        # "Folder exists\ndo nothing"
                      }
                    }
                    n127 = case shown="False" w183 {
                      tunnel: w181 -> [w213 _]
                      tunnel: w158 -> [w212 w214]
                      tunnel: [w212 w214] -> w156
                      frame False {
                        # "new folder"
                        n128 = Create Folder(path (use dialog)=w213) -> ()  [unwired: 2 in, 3 out]
                      }
                      frame True {
                        # "Folder exists\ndo nothing"
                      }
                    }
                    n129 = Concatenate Strings(w156, "\\Online_Raw_Data.dat" ("string")) -> (w175:string)
                    n130 = Concatenate Strings(w156, "\\Offline_Raw_Data.dat" ("string")) -> (w174:string)
                    n131 = Concatenate Strings(w155, "\\Online_Raw_Data.dat" ("string")) -> (w180:string)
                    n132 = Concatenate Strings(w155, "\\Offline_Raw_Data.dat" ("string")) -> (w179:string)
                    n133 = local read "DataOpen"() -> (w172:bool)
                    n134 = String To Path(string=w180) -> (path=w171:path)
                    n135 = String To Path(string=w179) -> (path=w170:path)
                    n136 = String To Path(string=w175) -> (path=w169:path)
                    n137 = String To Path(string=w174) -> (path=w168:path)
                    n138 = case shown="True" w172 {
                      tunnel: w171 -> [w203 w207]
                      tunnel: [w203 w207] -> w165
                      tunnel: w170 -> [w202 w206]
                      tunnel: [w202 w206] -> w164
                      tunnel: w169 -> [w201 w205]
                      tunnel: [w201 w205] -> w163
                      tunnel: [w200 w204] -> w162
                      tunnel: w168 -> [w200 w204]
                      frame False {
                        # "No files open\ndo nothing"
                      }
                      frame True {
                        # "Close open files"
                        n139 = local read "NF_Off_Ref"() -> (w209:refnum<file>)
                        n140 = local read "NF_On_Ref"() -> (w208:refnum<file>)
                        n141 = local read "FF_Off_Ref"() -> (w211:refnum<file>)
                        n142 = local read "FF_On_Ref"() -> (w210:refnum<file>)
                        n143 = Close File(refnum=w210) -> ()  [unwired: 1 in, 2 out]
                        n144 = Close File(refnum=w211) -> ()  [unwired: 1 in, 2 out]
                        n145 = Close File(refnum=w208) -> ()  [unwired: 1 in, 2 out]
                        n146 = Close File(refnum=w209) -> ()  [unwired: 1 in, 2 out]
                      }
                    }
                    n147 = Open/Create/Replace File(file path (use dialog)=w165, operation (0:open)=T7."open or create") -> (refnum out=w151:refnum<file>)  [unwired: 4 in, 2 out]
                    n148 = Open/Create/Replace File(file path (use dialog)=w164, operation (0:open)=T7."open or create") -> (refnum out=w152:refnum<file>)  [unwired: 4 in, 2 out]
                    n149 = Open/Create/Replace File(file path (use dialog)=w163, operation (0:open)=T7."open or create") -> (refnum out=w153:refnum<file>)  [unwired: 4 in, 2 out]
                    n150 = Open/Create/Replace File(file path (use dialog)=w162, operation (0:open)=T7."open or create") -> (refnum out=w154:refnum<file>)  [unwired: 4 in, 2 out]
                    n151 = Get File Size(file=w151) -> (refnum out=→"FF_On_Ref":refnum<file>, size (in bytes)=→"FF_On_Ptr":i64)  [unwired: 1 in, 1 out]
                    n152 = Get File Size(file=w152) -> (refnum out=→"FF_Off_Ref":refnum<file>, size (in bytes)=→"FF_Off_Ptr":i64)  [unwired: 1 in, 1 out]
                    n153 = Get File Size(file=w153) -> (refnum out=→"NF_On_Ref":refnum<file>, size (in bytes)=→"NF_On_Ptr":i64)  [unwired: 1 in, 1 out]
                    n154 = Get File Size(file=w154) -> (refnum out=→"NF_Off_Ref":refnum<file>, size (in bytes)=→"NF_Off_Ptr":i64)  [unwired: 1 in, 1 out]
                  }
                  frame True {
                    # "Don't need to do anything!"
                  }
                }
              }
              frame #1 {
                # "Writing and plotting retrieved\nweather parameters"
                # "Matlab script goes online and retrieves most recent press, temp, and relative humidity data \nfrom the weather station on the roof of Cobleigh"
                # "Importing the current weather conditions from the COE weather station"
                n155 = disable-structure shown="Disabled" {
                  frame Disabled {
                    n156 = script code="%try\n%s=urlread('http://www.coe.montana.edu/ee/weather/mostCurrentCSV.php');\n%amin=textscan(s,'%s %s %s %s %s %s %s %s %s %s %s %s %s');\n%data=amin{1}{2};\n%[test remain]=strtok(data,',');\n%remain=str2num(remain);\n%press=remain(3)./1000;\n%temp=remain(5);\n%RH=remain(7);\n%catch\npress=.850;\ntemp=20;\nRH=40;\n%end"() -> ()  [unwired: 1 in, 4 out]
                  }
                  frame Enabled {
                  }
                }
                "Temperature (C)" <- "Temperature (C)"
                "Pressure (mb)" <- "Pressure (mbar or hPa)"
                "Relative Humdity (%)" <- 40.0 ("Real")
              }
              frame #2 {
                # "Frame 3: Read, process, and plot online data\nFrame 4:\nFrame 5: Write the data to the folders from Frame 0 of outter sequence"
                # "Frame 0: Read the online wavelength and adjust to locking tolerance if out of range, Switch to offline DBR\nFrame 1: Read the output power from the Newport meter, calculate and plot the output pulse energy\nFrame 2: Wait 'Scalar Wait Time' for buffer to clear other wavelength data"
                # "Online"
                n157 = stacked-sequence {
                  frame #0 {
                    n158 = local read "L_Count"() -> (w235:i32)
                    n159 = Add(x=w235, y=60) -> (x+y=w233:i32)
                    n160 = Quotient & Remainder(x=w233, y=1.0) -> (x-y*floor(x/y)=w237:dbl)  [unwired: 1 out]
                    n161 = Equal To 0?(x=w237) -> (x = 0?=w236:bool)
                    n162 = case shown="True" w236 {
                      frame False {
                      }
                      frame True {
                        # "Read the online wavelength and continue adjusting the online DBR if outside the wavelength tolerance\nuntil it is within tolerance"
                        n163 = flat-sequence {
                          frame #0 {
                            # "Set the TSOA switch to\namplify the ABSORBING\nwavelength"
                            n164 = Build Array(FALSE ("Boolean")) -> (w239:bool[])
                            n165 = call-poly <vilib>:"DAQmx Write.vi"("task/channels in"=refnum<k21> "BristolWM", "data"=w239) -> ()  [unwired: 11 in, 3 out]
                          }
                          frame #1 {
                            n166 = while {
                              stop <- w242 stop-if-true
                              # "If WL difference is within tolerance, stop looping, and illuminate 'Wavelength Lock Online' indicator"
                              # "Frame 2: Decrement DBR current if above tolerance\nFrame 3: Increment DBR current if below tolerance"
                              # "Frame 0: Read the current wavelength from the wavemeter\nFrame 1: Calculate the difference between desired and actual wavelength"
                              # "Continue reading and adjusting online DBR current until within locking tolerance"
                              n167 = local read "AB_DIF"() -> (w245:dbl)
                              n168 = local read "ILX Address On"() -> (w243:dbl)
                              n169 = stacked-sequence {
                                tunnel: w243 -> [_ _ w257 w274]
                                frame #0 {
                                # "Reading the wavelength from the wavemeter"
                                n170 = flat-sequence {
                                frame #0 {
                                n171 = local read "Bristol In"() -> (w250:i32)
                                n172 = dll-call lib="C:/Users/H2ODial/Desktop/Shared Telescope WV DIAL Code/Libraries and VIs/CLDevIface.dll" fn="CLOpenUSBSerialDevice"("commPort"=w250) -> ("return type"=w249:i32)  [unwired: 4 in, 2 out]
                                n173 = local write "Bristol Out"(w249) -> ()
                                }
                                frame #1 {
                                n174 = local read "Bristol Out"() -> (w251:i32)
                                n175 = dll-call lib="C:/Users/H2ODial/Desktop/Shared Telescope WV DIAL Code/Libraries and VIs/CLDevIface.dll" fn="CLGetLambdaReading"("devHandle"=w251) -> ("return type"=→"Lambda On Read (nm)":dbl)  [unwired: 4 in, 2 out]
                                }
                                frame #2 {
                                n176 = local read "Bristol Out"() -> (w253:i32)
                                n177 = dll-call lib="C:/Users/H2ODial/Desktop/Shared Telescope WV DIAL Code/Libraries and VIs/CLDevIface.dll" fn="CLCloseDevice"("devHandle"=w253) -> ()  [unwired: 5 in, 2 out]
                                }
                                }
                                }
                                frame #1 {
                                # "Calculating the difference between the actual and desired online wavelength"
                                n178 = local read "Lambda On Read (nm)"() -> (w256:dbl)
                                n179 = Subtract(x=w256, y="Lambda On Set (nm)") -> (x-y=→"AB_DIF":dbl)
                                }
                                frame #2 {
                                # "If the wavelength difference is greater that 0.0002 nm, decrement the \nDBR current by 0.01 mA"
                                n180 = local read "AB_DIF"() -> (w260:dbl)
                                n181 = Greater Or Equal?(x=w260, y=0.0001) -> (x >= y?=w258:bool)
                                n182 = case shown="True" w258 {
                                tunnel: w257 -> [_ w261]
                                frame False {
                                # "Wavelength difference is not greater than 0.0002 nm, do nothing"
                                }
                                frame True {
                                n183 = stacked-sequence {
                                tunnel: w261 -> [w262 w265]
                                frame #0 {
                                # "Specifying laser channel 1,\nwhich is the online channel"
                                n184 = Number To Decimal String(number=w262) -> (decimal integer string=w263:string)  [unwired: 1 in]
                                n185 = GPIB Write(0:w263, 1:"LAS:CHAN 2") -> ()  [unwired: 3 in, 2 out]
                                }
                                frame #1 {
                                # "issuing the command"
                                # "Generating a command string\nto decrement the current"
                                # "WL difference is greater than 0.0002 nm,\ndecrement the DBR current by 0.01 mA"
                                n186 = local read "Lambda On DBR Current"() -> (w272:dbl)
                                n187 = Subtract(x=w272, y=0.01) -> (x-y=w266:dbl)
                                n188 = local write "Lambda On DBR Current"(w266) -> ()
                                n189 = Format Into String(format string="%.4f" ("Format String"), w266) -> (resulting string=w269:string)  [unwired: 2 in, 1 out]
                                n190 = Concatenate Strings("LAS:LDI ", w269) -> (w268:string)
                                n191 = Number To Decimal String(number=w265) -> (decimal integer string=w267:string)  [unwired: 1 in]
                                n192 = GPIB Write(0:w267, 1:w268) -> ()  [unwired: 3 in, 2 out]
                                }
                                }
                                }
                                }
                                }
                                frame #3 {
                                # "If WL difference is < 0.0002 nm, increment the DBR current"
                                n193 = local read "AB_DIF"() -> (w277:dbl)
                                n194 = Less Or Equal?(x=w277, y=-0.0001) -> (x <= y?=w275:bool)
                                n195 = case shown="True" w275 {
                                tunnel: w274 -> [_ w278]
                                frame False {
                                # "WL difference is no <= to -0.0002 nm, do nothing"
                                }
                                frame True {
                                n196 = stacked-sequence {
                                tunnel: w278 -> [w280 w282]
                                frame #0 {
                                # "Specifying laser channel 1,\nwhich is the online channel"
                                n197 = Number To Decimal String(number=w280) -> (decimal integer string=w279:string)  [unwired: 1 in]
                                n198 = GPIB Write(0:w279, 1:"LAS:CHAN 2") -> ()  [unwired: 3 in, 2 out]
                                }
                                frame #1 {
                                # "issuing the command"
                                # "Generating a command \nstring to increment the current"
                                # "WL difference is < -0.0002,\nincrement the DBR current by 0.01 mA"
                                n199 = local read "Lambda On DBR Current"() -> (w289:dbl)
                                n200 = Add(x=w289, y=0.01) -> (x+y=w284:dbl)
                                n201 = local write "Lambda On DBR Current"(w284) -> ()
                                n202 = Format Into String(format string="%.4f" ("Format String"), w284) -> (resulting string=w286:string)  [unwired: 2 in, 1 out]
                                n203 = Concatenate Strings("LAS:LDI ", w286) -> (w285:string)
                                n204 = Number To Decimal String(number=w282) -> (decimal integer string=w283:string)  [unwired: 1 in]
                                n205 = GPIB Write(0:w283, 1:w285) -> ()  [unwired: 3 in, 2 out]
                                }
                                }
                                }
                                }
                                }
                              }
                              n206 = Greater?(x=w245, y=-0.00011) -> (0:w247:bool)
                              n207 = Less?(x=w245, y=0.00011) -> (x < y?=w246:bool)
                              n208 = And(x=w247, y=w246) -> (x .and. y?=w242:bool)
                              "Wavelength Lock Online" <- w242
                            }
                          }
                          frame #2 {
                          }
                        }
                      }
                    }
                  }
                  frame #1 {
                    # "Converting to pulse energy, assumes 5 percent pickoff"
                    # "Reading the Newport Power meter"
                    # "Reading the output power of the laser transmitter from the Newport power meter, once read, convert to corresponding pulse energy and plot"
                    n209 = local read "Newport Device Key"() -> (w295:string)
                    n210 = local read "NewportRef"() -> (w291:refnum<k24>)
                    n211 = disable-structure shown="Disabled" {
                      frame Disabled {
                        # "Plotting the online and offling pulse energies"
                        n212 = local read "Online Pulse Energy"() -> (w306:dbl)
                        n213 = local read "Offline Pulse Energy"() -> (w305:dbl)
                        n214 = Bundle("Online Pulse Energy"=w306, "Offline Pulse Energy"=w305) -> (→"Pulse Energy (Micro Joule)":T9)  [unwired: 1 in]
                      }
                      frame Enabled {
                      }
                    }
                    n215 = Number To Decimal String(number="SampleSize") -> (decimal integer string=w293:string)  [unwired: 1 in]
                    n216 = invoke class="PowerMeterCommands" method="PerformDAQ"(reference=w291, "deviceKey"=w295, "interval"="1", "sampleSize"=w293) -> ("PerformDAQ"=w296:dbl[])  [unwired: 2 in, 5 out]
                    n217 = call-poly <vilib>:"Mean.vi"("X"=w296) -> ("mean"=w294:dbl)  [unwired: 1 out]
                    n218 = Multiply(x=w294, y=1000.0) -> (x*y=w302:dbl)
                    n219 = Divide(x=w302, y=0.05) -> (x/y=w300:dbl)
                    n220 = Divide(x=w300, y=7.0) -> (x/y=→"Online Pulse Energy":dbl)
                  }
                  frame #2 {
                    # "Waiting 'Scalar Wait Time'"
                    # "Wait 'Scalar Wait Time' for the next available batch of scalar card data"
                    n221 = Wait (ms)(milliseconds to wait="Scalar Wait Time") -> ()  [unwired: 1 out]
                  }
                  frame #3 {
                    # "convert time per range bin to meters\nand calculate smoothed bins using\nsmoothing range"
                    # "Plotting online cross section and smoothed online data"
                    # "Calculate the bin by bin mean of the data"
                    # "Collect 'Integration Period (Seconds)' number\nof scalar data"
                    # "Reading, processing, and plotting the online data"
                    n222 = local read "Data Reads (number of loops)"() -> (w333:i32)
                    n223 = for {
                      N: w333 -> [_]
                      tunnel: [w354] -> w345 mode=indexing
                      tunnel: [w353] -> w308 mode=indexing
                      # "Scalar Data is retrieved from Global \nVariable that scaler.vi is writing to,"
                      n224 = global read "Scalar_Data.vi" "Scalar Data"() -> (w354:u16[])
                      n225 = global read "Scalar_Data_3.vi" "Scalar Data 3"() -> (w353:u16[])
                    }
                    n226 = Transpose 2D Array(2D array=w345) -> (transposed array=w349:u16[][])
                    n227 = Transpose 2D Array(2D array=w308) -> (transposed array=w331:u16[][])
                    n228 = for {
                      tunnel: w349 -> [w356] mode=indexing
                      tunnel: [w355] -> w350 mode=indexing
                      n229 = call-poly <vilib>:"Mean.vi"("X"=w356) -> ("mean"=w355:dbl)  [unwired: 1 out]
                    }
                    n230 = for {
                      tunnel: w331 -> [w352] mode=indexing
                      tunnel: [w351] -> w332 mode=indexing
                      n231 = call-poly <vilib>:"Mean.vi"("X"=w352) -> ("mean"=w351:dbl)  [unwired: 1 out]
                    }
                    n232 = local read "bins"() -> (w325:u32)
                    n233 = Array Subset(array=w350, index=1 ("dimension size"), length=w325) -> (w337:dbl[])
                    n234 = Array Subset(array=w332, index=1 ("dimension size"), length=w325) -> (w329:dbl[])
                    n235 = local read "background length"() -> (w315:i32)
                    n236 = local read "background start"() -> (w316:u32)
                    n237 = Array Size(array=w337) -> (size(s)=w334:i32)
                    n238 = Array Size(array=w329) -> (size(s)=w326:i32)
                    n239 = Initialize Array(1.0 ("element"), w334) -> (w336:dbl[])
                    n240 = Initialize Array(1.0 ("element"), w326) -> (w328:dbl[])
                    n241 = Multiply(x=w337, y=w336) -> (x*y=w338:dbl[])
                    "On-Line Bin Readings" <- w338
                    n242 = Multiply(x=w329, y=w328) -> (x*y=w319:dbl[])
                    "On-Line Bin Readings 2" <- w319
                    n243 = local read "Total DIAL Integration Time (Minutes)"() -> (w341:i32)
                    n244 = local read "Time Resolution Per Bin(ns)"() -> (w311:u32)
                    n245 = Array Subset(array=w338, index=w316, length=w315) -> (w347:dbl[])
                    n246 = Array Subset(array=w319, index=w316, length=w315) -> (w321:dbl[])
                    n247 = call-poly <vilib>:"Mean.vi"("X"=w347) -> ("mean"=w346:dbl)  [unwired: 1 out]
                    n248 = call-poly <vilib>:"Mean.vi"("X"=w321) -> ("mean"=w322:dbl)  [unwired: 1 out]
                    n249 = Divide(x=w341, y=w333) -> (x/y=w339:dbl)
                    n250 = local read "Index"() -> (w320:i32)
                    n251 = Subtract(x=w338, y=w346) -> (x-y=w343:dbl[])
                    n252 = Subtract(x=w319, y=w322) -> (x-y=w323:dbl[])
                    n253 = To Double Precision Float(number=w311) -> (double precision float=w312:dbl)
                    n254 = Multiply(x=w339, y=60.0) -> (x*y=w317:dbl)
                    n255 = Multiply(x=w312, y=0.15) -> (x*y=w314:dbl)
                    n256 = call "Ring Buffer Online Far.vi"("Index"=w320, "Profiles to Average"=w317, "Input Array"=w343) -> ("AvgArray"=w342:dbl[])  [unwired: 7 in, 1 out]
                    n257 = call "Ring Buffer Online Near.vi"("Index"=w320, "Profiles to Average"=w317, "Input Array"=w323) -> ("AvgArray"=w324:dbl[])  [unwired: 7 in, 1 out]
                    n258 = Divide(x="Smoothing Range", y=w314) -> (x/y=w309:dbl)
                    "Smoothed Bins" <- w309
                    n259 = call "Smooth Arrray.vi"("smooth size"=w309, "Raw Array"=w342) -> ("Smoothed Array"=→"On-Line  Smoothed":dbl[])  [unwired: 9 in]
                    n260 = call "Smooth Arrray.vi"("smooth size"=w309, "Raw Array"=w324) -> ("Smoothed Array"=→"On-Line Smoothed 2":dbl[])  [unwired: 9 in]
                    n261 = disable-structure shown="Disabled" {
                      frame Disabled {
                        n262 = script code="format long;\ncounts=sum(Online);\nif counts >=0.5e6\ntime=time;\nelse\ntime=time\nend"() -> ()  [unwired: 3 in, 2 out]
                      }
                      frame Enabled {
                      }
                    }
                  }
                  frame #4 {
                    # "Toggling the Agiltron switch to the offline DBR seed laser"
                    n263 = disable-structure shown="Disabled" {
                      frame Disabled {
                        n264 = flat-sequence {
                          frame #0 {
                            # "Second one"
                            # "Command the switch to switch to position 2\ncorresponding to the offline DBR"
                            # "Hex string command \ncorrespond to offline"
                            n265 = VISA Write(VISA resource name="Switch Comm Port", write buffer="\u0001\u0012\u0000\u0001") -> ()  [unwired: 1 in, 3 out]
                          }
                        }
                      }
                      frame Enabled {
                      }
                    }
                  }
                  frame #5 {
                    # "Save the recently collected online data if 'Save Data?' is true"
                    n266 = case shown="True" "Save Data?" {
                      frame False {
                        # "'Save Data?' is false, do nothing"
                      }
                      frame True {
                        # "'Save Data?' is true, save onfline data to the Data Disk"
                        # "Write only one copy of data at this time"
                        # "Retrieve Julian Date"
                        n267 = local read "Lambda On DBR Current"() -> (w384:dbl)
                        n268 = local read "Lambda On Read (nm)"() -> (w385:dbl)
                        n269 = local read "On-Line Bin Readings 2"() -> (w379:dbl[])
                        n270 = local read "Relative Humdity (%)"() -> (w380:dbl)
                        n271 = local read "On-Line Bin Readings"() -> (w387:dbl[])
                        n272 = local read "Online Pulse Energy"() -> (w383:dbl)
                        n273 = local read "Temperature (C)"() -> (w382:dbl)
                        n274 = local read "Pressure (mb)"() -> (w381:dbl)
                        n275 = call "Julian_Date_2.vi"() -> ("Julian Date"=w386:dbl)  [unwired: 11 in]
                        n276 = Build Array (concatenate)(w386, w385, w384, w383, w382, w381, w380, w387) -> (w374:dbl[])
                        n277 = Build Array (concatenate)(w386, w385, w384, w383, w382, w381, w380, w379) -> (w364:dbl[])
                        n278 = local write "DataOpen"(TRUE ("DataOpen")) -> ()
                        n279 = local read "NF_On_Ref"() -> (w362:refnum<file>)
                        n280 = local read "FF_On_Ref"() -> (w378:refnum<file>)
                        n281 = local read "NF_On_Ptr"() -> (w363:i64)
                        n282 = local read "FF_On_Ptr"() -> (w377:i64)
                        n283 = Set File Position(offset (in bytes) (0)=w377, refnum=w378) -> (refnum out=w375:refnum<file>, error out=w372:errorcluster)  [unwired: 2 in]
                        n284 = Set File Position(offset (in bytes) (0)=w363, refnum=w362) -> (refnum out=w368:refnum<file>, error out=w366:errorcluster)  [unwired: 2 in]
                        n285 = Write to Binary File(file (use dialog)=w368, data=w364, error in=w366, 5:FALSE ("prepend array or string size? (T)")) -> (refnum out=w367:refnum<file>, error out=w365:errorcluster)  [unwired: 2 in, 1 out]
                        n286 = Write to Binary File(file (use dialog)=w375, data=w374, error in=w372, 5:FALSE ("prepend array or string size? (T)")) -> (refnum out=w373:refnum<file>, error out=w371:errorcluster)  [unwired: 2 in, 1 out]
                        n287 = Get File Position(4:w365, 7:w367) -> (2:w361:i64)  [unwired: 2 out]
                        n288 = Get File Position(4:w371, 7:w373) -> (2:w370:i64)  [unwired: 2 out]
                        n289 = local write "NF_On_Ptr"(w361) -> ()
                        n290 = local write "FF_On_Ptr"(w370) -> ()
                      }
                    }
                  }
                }
              }
              frame #3 {
                # "Frame 3: Read offline data, calculate aerosol data, and plot offline and normalized relative backscatter\nFrame 4:\nFrame 5: Save the offline data and related information"
                # "Frame 0: Read the offline wavelength and lock if necessary, Switch to online DBR\nFrame 1: Read the output power from the Newport power meter\nFrame 2: Wait 'Scalar Wait Time' for buffers to clear of online contiminated data"
                # "offline"
                n291 = stacked-sequence {
                  frame #0 {
                    # "Every 60 data collection cycles, read the offline DBR wavelength, and if outside of wavelength tolerance, adjust DBR current until within tolerance"
                    n292 = local read "L_Count"() -> (w389:i32)
                    n293 = Quotient & Remainder(x=w389, y=60.0) -> (x-y*floor(x/y)=w390:dbl)  [unwired: 1 out]
                    n294 = Equal To 0?(x=w390) -> (x = 0?=w388:bool)
                    n295 = case shown="True" w388 {
                      frame False {
                      }
                      frame True {
                        n296 = flat-sequence {
                          frame #0 {
                            # "Set the TSOA switch to\namplify the non ABSORBING\nwavelength"
                            n297 = Build Array(TRUE ("Boolean")) -> (w392:bool[])
                            n298 = call-poly <vilib>:"DAQmx Write.vi"("task/channels in"=refnum<k21> "BristolWM", "data"=w392) -> ()  [unwired: 11 in, 3 out]
                          }
                          frame #1 {
                            n299 = while {
                              stop <- w395 stop-if-true
                              # "If WL difference is within tolerance, stop looping, and illuminate 'Wavelength Lock Offline' indicator"
                              # "Frame 2: Decrement DBR current if above tolerance\nFrame 3: Increment DBR current if below tolerance"
                              # "Frame 0: Read the current wavelength from the wavemeter\nFrame 1: Calculate the difference between desired and actual wavelength"
                              # "Continue reading and adjusting offline DBR current until within locking tolerance"
                              n300 = local read "NONAB_DIF"() -> (w398:dbl)
                              n301 = local read "ILX Address Off"() -> (w396:dbl)
                              n302 = stacked-sequence {
                                tunnel: w396 -> [_ _ w410 w427]
                                frame #0 {
                                # "Reading the wavelength from the wavemeter"
                                n303 = flat-sequence {
                                frame #0 {
                                n304 = local read "Bristol In"() -> (w403:i32)
                                n305 = dll-call lib="C:/Users/H2ODial/Desktop/Shared Telescope WV DIAL Code/Libraries and VIs/CLDevIface.dll" fn="CLOpenUSBSerialDevice"("commPort"=w403) -> ("return type"=w402:i32)  [unwired: 4 in, 2 out]
                                n306 = local write "Bristol Out"(w402) -> ()
                                }
                                frame #1 {
                                n307 = local read "Bristol Out"() -> (w405:i32)
                                n308 = dll-call lib="C:/Users/H2ODial/Desktop/Shared Telescope WV DIAL Code/Libraries and VIs/CLDevIface.dll" fn="CLGetLambdaReading"("devHandle"=w405) -> ("return type"=→"Lambda Off Read (nm)":dbl)  [unwired: 4 in, 2 out]
                                }
                                frame #2 {
                                n309 = local read "Bristol Out"() -> (w406:i32)
                                n310 = dll-call lib="C:/Users/H2ODial/Desktop/Shared Telescope WV DIAL Code/Libraries and VIs/CLDevIface.dll" fn="CLCloseDevice"("commPort"=w406) -> ()  [unwired: 5 in, 2 out]
                                }
                                }
                                }
                                frame #1 {
                                # "Calculating the difference between the actual and desired online wavelength"
                                n311 = local read "Lambda Off Read (nm)"() -> (w409:dbl)
                                n312 = Subtract(x=w409, y="Lambda Off Set (nm)") -> (x-y=→"NONAB_DIF":dbl)
                                }
                                frame #2 {
                                # "If the wavelength difference is greater that 0.0002 nm, decrement the \nDBR current by 0.01 mA"
                                n313 = local read "NONAB_DIF"() -> (w413:dbl)
                                n314 = Greater Or Equal?(x=w413, y=0.0001) -> (x >= y?=w411:bool)
                                n315 = case shown="True" w411 {
                                tunnel: w410 -> [_ w414]
                                frame False {
                                # "Wavelength difference is not greater than 0.0002 nm, do nothing"
                                }
                                frame True {
                                n316 = stacked-sequence {
                                tunnel: w414 -> [w415 w418]
                                frame #0 {
                                # "Specifying laser channel 1,\nwhich is the online channel"
                                n317 = Number To Decimal String(number=w415) -> (decimal integer string=w416:string)  [unwired: 1 in]
                                n318 = GPIB Write(0:w416, 1:"LAS:CHAN 2") -> ()  [unwired: 3 in, 2 out]
                                }
                                frame #1 {
                                # "issuing the command"
                                # "Generating a command string\nto decrement the current"
                                # "WL difference is greater than 0.0002 nm,\ndecrement the DBR current by 0.01 mA"
                                n319 = local read "Lambda Off DBR Current"() -> (w425:dbl)
                                n320 = Subtract(x=w425, y=0.01) -> (x-y=w419:dbl)
                                n321 = local write "Lambda Off DBR Current"(w419) -> ()
                                n322 = Format Into String(format string="%.4f" ("Format String"), w419) -> (resulting string=w422:string)  [unwired: 2 in, 1 out]
                                n323 = Concatenate Strings("LAS:LDI ", w422) -> (w421:string)
                                n324 = Number To Decimal String(number=w418) -> (decimal integer string=w420:string)  [unwired: 1 in]
                                n325 = GPIB Write(0:w420, 1:w421) -> ()  [unwired: 3 in, 2 out]
                                }
                                }
                                }
                                }
                                }
                                frame #3 {
                                # "If WL difference is < 0.0002 nm, increment the DBR current"
                                n326 = local read "NONAB_DIF"() -> (w430:dbl)
                                n327 = Less Or Equal?(x=w430, y=-0.0001) -> (x <= y?=w428:bool)
                                n328 = case shown="True" w428 {
                                tunnel: w427 -> [_ w431]
                                frame False {
                                # "WL difference is no <= to -0.0002 nm, do nothing"
                                }
                                frame True {
                                n329 = stacked-sequence {
                                tunnel: w431 -> [w433 w435]
                                frame #0 {
                                # "Specifying laser channel 1,\nwhich is the online channel"
                                n330 = Number To Decimal String(number=w433) -> (decimal integer string=w432:string)  [unwired: 1 in]
                                n331 = GPIB Write(0:w432, 1:"LAS:CHAN 2") -> ()  [unwired: 3 in, 2 out]
                                }
                                frame #1 {
                                # "issuing the command"
                                # "Generating a command \nstring to increment the current"
                                # "WL difference is < -0.0002,\nincrement the DBR current by 0.01 mA"
                                n332 = local read "Lambda Off DBR Current"() -> (w442:dbl)
                                n333 = Add(x=w442, y=0.01) -> (x+y=w437:dbl)
                                n334 = local write "Lambda Off DBR Current"(w437) -> ()
                                n335 = Format Into String(format string="%.4f" ("Format String"), w437) -> (resulting string=w439:string)  [unwired: 2 in, 1 out]
                                n336 = Concatenate Strings("LAS:LDI ", w439) -> (w438:string)
                                n337 = Number To Decimal String(number=w435) -> (decimal integer string=w436:string)  [unwired: 1 in]
                                n338 = GPIB Write(0:w436, 1:w438) -> ()  [unwired: 3 in, 2 out]
                                }
                                }
                                }
                                }
                                }
                              }
                              n339 = Greater?(x=w398, y=-0.00011) -> (0:w400:bool)
                              n340 = Less?(x=w398, y=0.00011) -> (x < y?=w399:bool)
                              n341 = And(x=w400, y=w399) -> (x .and. y?=w395:bool)
                              "Wavelength Lock Offline" <- w395
                            }
                          }
                          frame #2 {
                            # "Set the TSOA switch to\namplify the ABSORBING\nwavelength"
                            n342 = Build Array(FALSE ("Boolean")) -> (w444:bool[])
                            n343 = call-poly <vilib>:"DAQmx Write.vi"("task/channels in"=refnum<k21> "BristolWM", "data"=w444) -> ()  [unwired: 11 in, 3 out]
                          }
                        }
                      }
                    }
                  }
                  frame #1 {
                    # "Reading the power meter"
                    # "Updating the pulse energy plot"
                    # "Converting to pulse energy"
                    # "Reading the offline output power, converting to pulse energy,  and updating the Pulse energy plot"
                    n344 = local read "SampleSize"() -> (w449:i32)
                    n345 = local read "Newport Device Key"() -> (w450:string)
                    n346 = local read "Online Pulse Energy"() -> (w456:dbl)
                    n347 = local read "Offline Pulse Energy"() -> (w455:dbl)
                    n348 = local read "NewportRef"() -> (w447:refnum<k24>)
                    n349 = Number To Decimal String(number=w449) -> (decimal integer string=w451:string)  [unwired: 1 in]
                    n350 = invoke class="PowerMeterCommands" method="PerformDAQ"(reference=w447, "deviceKey"=w450, "interval"="1", "sampleSize"=w451) -> ("PerformDAQ"=w452:dbl[])  [unwired: 2 in, 5 out]
                    n351 = Bundle("Online Pulse Energy"=w456, "Offline Pulse Energy"=w455) -> (w454:T9)  [unwired: 1 in]
                    n352 = local write "Pulse Energy (Micro Joule)"(w454) -> ()
                    n353 = call-poly <vilib>:"Mean.vi"("X"=w452) -> ("mean"=w448:dbl)  [unwired: 1 out]
                    n354 = Multiply(x=w448, y=1000.0) -> (x*y=w461:dbl)
                    n355 = Divide(x=w461, y=0.05) -> (x/y=w459:dbl)
                    n356 = Divide(x=w459, y=7.0) -> (x/y=→"Offline Pulse Energy":dbl)
                  }
                  frame #2 {
                    # "Wait 'Scalar Wait Time' for buffers to clear of online contiminated offline data"
                    n357 = disable-structure shown="Disabled" {
                      frame Disabled {
                        # "Wait 'Scalar Wait Time'"
                        n358 = local read "Scalar Wait Time"() -> (w463:u32)
                        n359 = Wait (ms)(milliseconds to wait=w463) -> ()  [unwired: 1 out]
                      }
                      frame Enabled {
                      }
                    }
                  }
                  frame #3 {
                    w497 = 1 ("dimension size")
                    w501 = 1
                    # "Plotting the normalized relative \nbackscatter"
                    # "Calculating the normalized relative backscatter"
                    # "Calculating/Plotting smoothed data,\ncross sections etc."
                    # "Pick off data with\nout header"
                    # "Calculate mean bin by bin mean"
                    # "Reading in 'Integration Period (Seconds)' of data"
                    # "Read the offline data from the scalar card, perform smoothing, calculate normalized relative backscatter, and plot"
                    # "File path in MATLAB script is of old dial is:\nF:\\Micropulse DIAL\\Micropulse DIAL Matlab\\\nFinal Overlap Function.mat')];"
                    # "Collects Data From Card,\nSends It To The Chart,\nAnd Saves A Copy As A\nFile If Option Selected On\nFront Panel"
                    n360 = for {
                      N: "Data Reads (number of loops)" -> [_]
                      tunnel: [w533] -> w465 mode=indexing
                      tunnel: [w532] -> w464 mode=indexing
                      # "Read in latest scalar card data from \n'Scalar Data' global variable that \nscaler.vi is writing to, then wait 1 sec\nfor next batch of data"
                      n361 = global read "Scalar_Data_2.vi" "Scalar Data 2"() -> (w533:u16[])
                      n362 = global read "Scalar_Data_4.vi" "Scalar Data 4"() -> (w532:u16[])
                    }
                    n363 = local read "Total DIAL Integration Time (Minutes)"() -> (w522:i32)
                    n364 = Divide(x=w522, y="Data Reads (number of loops)") -> (x/y=w520:dbl)
                    n365 = local read "Total Aerosol Integration Time (Minutes)"() -> (w524:dbl)
                    n366 = local read "background length"() -> (w469:i32)
                    n367 = Multiply(x=w520, y=60.0) -> (x*y=w507:dbl)
                    n368 = local read "background start"() -> (w470:u32)
                    n369 = Transpose 2D Array(2D array=w465) -> (transposed array=w530:u16[][])
                    n370 = Transpose 2D Array(2D array=w464) -> (transposed array=w513:u16[][])
                    n371 = Divide(x=w524, y="Data Reads (number of loops)") -> (x/y=w525:dbl)
                    n372 = for {
                      tunnel: w530 -> [w537] mode=indexing
                      tunnel: [w536] -> w531 mode=indexing
                      tunnel: w513 -> [w535] mode=indexing
                      tunnel: [w534] -> _ mode=indexing
                      tunnel: [w534] -> w510 mode=indexing
                      n373 = call-poly <vilib>:"Mean.vi"("X"=w537) -> ("mean"=w536:dbl)  [unwired: 1 out]
                      n374 = call-poly <vilib>:"Mean.vi"("X"=w535) -> ("mean"=w534:dbl)  [unwired: 1 out]
                    }
                    n375 = local read "bins"() -> (w498:u32)
                    n376 = Multiply(x=w525, y=60.0) -> (x*y=w488:dbl)
                    n377 = Array Subset(array=w510, index=w497, length=w498) -> (w511:dbl[])
                    "Off-Line Bin Readings 2" <- w511
                    n378 = Array Subset(array=w531, index=w497, length=w498) -> (w509:dbl[])
                    "Off-Line  Bin Readings" <- w509
                    n379 = Array Subset(array=w511, index=w470, length=w469) -> (w512:dbl[])
                    n380 = Array Subset(array=w509, index=w470, length=w469) -> (w529:dbl[])
                    n381 = local read "Smoothed Bins"() -> (w466:dbl)
                    n382 = call-poly <vilib>:"Mean.vi"("X"=w512) -> ("mean"=w476:dbl)  [unwired: 1 out]
                    n383 = call-poly <vilib>:"Mean.vi"("X"=w529) -> ("mean"=w477:dbl)  [unwired: 1 out]
                    n384 = local read "Index"() -> (w487:i32)
                    n385 = Subtract(x=w511, y=w476) -> (x-y=w489:dbl[])
                    n386 = Subtract(x=w509, y=w477) -> (x-y=w505:dbl[])
                    n387 = call "Ring Buffer Offline Far.vi"("Index"=w487, "Profiles to Average"=w507, "Input Array"=w505) -> ("AvgArray"=w527:dbl[], "RingBufferOut"=→"RingBuffer offline far":dbl[][])  [unwired: 7 in]
                    n388 = call "Ring Buffer Aerosol Far.vi"("Index"=w487, "Profiles to Average"=w488, "Input Array"=w505) -> ("AvgArray"=w523:dbl[], "RingBufferOut"=→"RingBuffer aerosol far":dbl[][])  [unwired: 7 in]
                    n389 = call "Ring Buffer Offline Near.vi"("Index"=w487, "Profiles to Average"=w507, "Input Array"=w489) -> ("AvgArray"=w508:dbl[], "RingBufferOut"=→"RingBuffer offline near":dbl[][])  [unwired: 7 in]
                    n390 = call "Ring Buffer Aerosol Near.vi"("Index"=w487, "Profiles to Average"=w488, "Input Array"=w489) -> ("AvgArray"=w485:dbl[], "RingBufferOut"=→"RingBuffer aerosol near":dbl[][])  [unwired: 7 in]
                    n391 = Reshape Array(w505, w497, w498) -> (→"raw counts":dbl[][])
                    n392 = Reshape Array(w489, w497, w498) -> (→"raw counts near":dbl[][])
                    n393 = call "Smooth Arrray.vi"("smooth size"=w466, "Raw Array"=w527) -> ("Smoothed Array"=→"Off-Line Smoothed":dbl[])  [unwired: 9 in]
                    n394 = call "Smooth Arrray.vi"("smooth size"=w466, "Raw Array"=w523) -> ("Smoothed Array"=w496:dbl[])  [unwired: 9 in]
                    "Aerosol Smoothed" <- w496
                    n395 = call "Smooth Arrray.vi"("smooth size"=w466, "Raw Array"=w508) -> ("Smoothed Array"=→"Off-Line Smoothed 2":dbl[])  [unwired: 9 in]
                    n396 = call "Smooth Arrray.vi"("smooth size"=w466, "Raw Array"=w485) -> ("Smoothed Array"=w468:dbl[])  [unwired: 9 in]
                    "Aerosol Smoothed 2" <- w468
                    n397 = local read "Number of Accumulates"() -> (w472:u32)
                    n398 = local read "Temperature (C)"() -> (w519:dbl)
                    n399 = local read "Pressure (mb)"() -> (w518:dbl)
                    n400 = script code="%accum_num=10000;     % scaler card setting number of accumulations\nt_bin = 500e-9                 % scaler card setting time per bin\n%t_d = 37.3e-9;                % APD dead time from spec sheet\n\n% conversion from accumulated counts to count rate  (c/s)\nc_convert = 1./t_bin./accum_num;\nCR_far = p_raw_far.*c_convert;\nCR_near = p_raw_near.*c_convert;\nCR_total_far = (p_raw_far+b_far).*c_convert;\nCR_total_near = (p_raw_near+b_near).*c_convert;\nb_CR_far =b_far.*c_convert;\nb_CR_near =b_near.*c_convert;\n\n% create a range array\nsize_p =  size(p_raw_far,2);\nr = (75:75:size_p*75)./1e3; \n    \n%APD correction factor\n D_far = 1./(1-(t_d*CR_total_far));\n D_near = 1./(1-(t_d*CR_total_near));\n\n %Calculating normalize relative backscatter profile\n nrb_far = CR_far.*D_far.*r.^2./E.*1e-6;\n nrb_near = CR_near.*D_near.*r.^2./E.*1e-6;"("E"=6.0 ("Real"), "temp"=w519, "press"=w518, "p_raw_far"=w496, "b_far"=w477, "b_near"=w476, "p_raw_near"=w468, "accum_num"=w472, "t_d"="dead time") -> ("nrb_far"=w491:cdb[], "D_far"=w482:dbl[], "nrb_near"=w490:cdb[], "D_near"=w481:dbl[], "b_CR_far"=w474:dbl, "b_CR_near"=w473:dbl)  [unwired: 1 in, 1 out]
                    n401 = local read "bins"() -> (w500:u32)
                    n402 = local read "Altitude Array (km)"() -> (w493:dbl[])
                    n403 = Bundle(w474, w473) -> (→"?":cluster{dbl, dbl})  [unwired: 1 in]
                    n404 = Build Array(w491, w490) -> (w495:cdb[][])
                    n405 = Build Array(w482, w481) -> (w480:dbl[][])
                    n406 = Reshape Array(w490, w501, w500) -> (→"NRB 2":cdb[][])
                    n407 = Reshape Array(w491, w501, w500) -> (→"NRB":cdb[][])
                    n408 = Build Array(w493, w493) -> (w492:dbl[][])
                    n409 = call "Convert to Dynamic Data7"("2D Array"=w480) -> ("Dynamic Data Type"=w479:dynamicdata)  [unwired: 3 in]
                    n410 = call "Convert to Dynamic Data3"("2D Array"=w495) -> ("Dynamic Data Type"=w494:dynamicdata)  [unwired: 3 in]
                    n411 = call "Convert to Dynamic Data4"("2D Array"=w492) -> ("Dynamic Data Type"=w483:dynamicdata)  [unwired: 3 in]
                    n412 = call "Build XY Graph2"("Y Input"=w483, "X Input"=w494) -> ("XY Graph"=→"NRB plot":cluster{"Y":dbl[], "Y":dbl[]}[])  [unwired: 3 in, 6 out]
                    n413 = call "Build XY Graph4"("Y Input"=w483, "X Input"=w479) -> ("XY Graph"=→"Correction":cluster{"Y":dbl[], "Y":dbl[]}[])  [unwired: 3 in, 6 out]
                  }
                  frame #4 {
                    # "REPLACE WITH NEW AGILTRON TASK!"
                    # "Toggle Agiltron switch to online DBR"
                    n414 = disable-structure shown="Disabled" {
                      frame Disabled {
                        # "ABSORBING"
                        n415 = flat-sequence {
                          frame #0 {
                            # "Third one"
                            # "Command the switch to switch to position 1\ncorresponding to the online DBR"
                            # "Hex string command \ncorrespond to online"
                            n416 = local read "Switch Comm Port"() -> (w541:refnum<visa-resource-name>)
                            n417 = VISA Write(VISA resource name=w541, write buffer="\u0001\u0012\u0000\u0002") -> ()  [unwired: 1 in, 3 out]
                          }
                        }
                        n418 = Build Array(FALSE ("Boolean")) -> (w540:bool[])
                        n419 = call-poly <vilib>:"DAQmx Write.vi"("task/channels in"=refnum<k21> "AgiltronSwitch", "data"=w540) -> ()  [unwired: 11 in, 3 out]
                      }
                      frame Enabled {
                      }
                    }
                  }
                  frame #5 {
                    # "If 'Save Data?' is true, save all relavant offline info"
                    n420 = local read "Save Data?"() -> (w543:bool)
                    n421 = case shown="True" w543 {
                      frame False {
                        # "'Save Data?' is false, do nothing"
                      }
                      frame True {
                        # "Write only one data file at this time"
                        # "Retrive Julian Date"
                        # "'Save Data?' is true, save offline data to the Data Disk"
                        n422 = local read "Lambda Off DBR Current"() -> (w565:dbl)
                        n423 = local read "Off-Line Bin Readings 2"() -> (w562:dbl[])
                        n424 = local read "Lambda Off Read (nm)"() -> (w564:dbl)
                        n425 = local read "Off-Line  Bin Readings"() -> (w570:dbl[])
                        n426 = local read "Relative Humdity (%)"() -> (w569:dbl)
                        n427 = local read "Offline Pulse Energy"() -> (w566:dbl)
                        n428 = local read "Temperature (C)"() -> (w567:dbl)
                        n429 = local read "Pressure (mb)"() -> (w568:dbl)
                        n430 = call "Julian_Date_2.vi"() -> ("Julian Date"=w563:dbl)  [unwired: 11 in]
                        n431 = Build Array (concatenate)(w563, w564, w565, w566, w567, w568, w569, w570) -> (w548:dbl[])
                        n432 = Build Array (concatenate)(w563, w564, w565, w566, w567, w568, w569, w562) -> (w545:dbl[])
                        n433 = local read "FF_Off_Ref"() -> (w550:refnum<file>)
                        n434 = local read "NF_Off_Ref"() -> (w547:refnum<file>)
                        n435 = local read "FF_Off_Ptr"() -> (w549:i64)
                        n436 = local read "NF_Off_Ptr"() -> (w546:i64)
                        n437 = Set File Position(offset (in bytes) (0)=w549, refnum=w550) -> (refnum out=w561:refnum<file>, error out=w559:errorcluster)  [unwired: 2 in]
                        n438 = Set File Position(offset (in bytes) (0)=w546, refnum=w547) -> (refnum out=w557:refnum<file>, error out=w555:errorcluster)  [unwired: 2 in]
                        n439 = Write to Binary File(file (use dialog)=w561, data=w548, error in=w559, 5:FALSE ("prepend array or string size? (T)")) -> (refnum out=w560:refnum<file>, error out=w558:errorcluster)  [unwired: 2 in, 1 out]
                        n440 = Write to Binary File(file (use dialog)=w557, data=w545, error in=w555, 5:FALSE ("prepend array or string size? (T)")) -> (refnum out=w556:refnum<file>, error out=w554:errorcluster)  [unwired: 2 in, 1 out]
                        n441 = Get File Position(4:w558, 7:w560) -> (2:w551:i64)  [unwired: 2 out]
                        n442 = Get File Position(4:w554, 7:w556) -> (2:w544:i64)  [unwired: 2 out]
                        n443 = local write "FF_Off_Ptr"(w551) -> ()
                        n444 = local write "NF_Off_Ptr"(w544) -> ()
                      }
                    }
                  }
                }
              }
              frame #4 {
                n445 = First Call?() -> (First Call?: T/F=w573:bool)
                n446 = Or(x="calculate absorption cross sections", y=w573) -> (x .or. y?=w571:bool)
                n447 = case shown="True" w571 {
                  frame False {
                  }
                  frame True {
                    # "calculate absorption cross sections from HITRAN data base"
                    n448 = local read "Off-Line Smoothed"() -> (w574:dbl[])
                    n449 = local read "Lambda On Read (nm)"() -> (w577:dbl)
                    n450 = local read "Lambda Off Set (nm)"() -> (w580:dbl)
                    n451 = local read "Temperature (C)"() -> (w578:dbl)
                    n452 = local read "Pressure (mb)"() -> (w579:dbl)
                    n453 = script code="%Importing HITRAN data\n%hitran = dlmread('C:\\Users\\H2ODial\\Desktop\\Shared Telescope WV DIAL Code\\Libraries and VIs\\824nm_841nm_H2O.csv', ',',[0 1 352 7]);\nhitran = dlmread('C:\\Users\\H2ODial\\Desktop\\Shared Telescope WV DIAL Code\\Libraries and VIs\\824nm_841nm_H2O_Spectral_Calc.csv', ',',[1 1 1209 7]);\n\n%Range vector in meters\nrange = ([75:75:size(Online,2)*75]);\n\nif lambda< 828\nlambda=828.195;\nelse\nlambda=lambda;\nend;\n\n%%\n\n%Voigt profile calculation\nWNmin = 12070.0;\nWNmax = 12076.0;\n\n%Find lines from WNmin to WNmax to calculate voigt profile\nline_indices = find(hitran(1:size(hitran,1),1)>WNmin & hitran(1:size(hitran,1),1)<WNmax);\n\nline = (hitran(line_indices, 1:size(hitran,2)));\n\n%Calculate temperature and pressure profile\nT0 = 273+15.6;\nT0 = 273+T0_C;\n\nT = T0-0.005545.*range; \n\nP0  = 1.0;\nP0  = P0_mb/1000*0.986; %pressure in mb converted to atm\n\nP = P0.*(T0./T).^-5.21986;\n\n%linewidth temperature dependence factor\nalpha = line(:,7);        \n\n%initial Lorentz linewidth from HiTRAN [cm^-1]\ngammal0 = line(:,4);     \n\n%ground state transition energy [cm^-1]\nE = line(:,6);           \n\n%initial linestrength from HiTRAN [cm^-1/(mol*cm^-2)]\nS0 = line(:,2);      \n\n%absorption line center wavenumber from HiTRAN [cm^-1]\nnu0_0 = line(:,1);    \n\nnu_on = (1/(lambda)*1e7);\n\nnu_off = (1/(lambda_off)*1e7);\n\n\nfor i = 1:size(Online,2);\n\n    %Pressure shift\n    nu0 = nu0_0-.0428.*P(i);\n    \n    %Calculate Lorentz lineweidth at temperature T [cm^-1]\n    gammal = gammal0.*(P(i)./P0).*((T0./T(i)).^alpha);\n    \n    %Calculate Doppler linewidth at temperature T [cm^-1]\n    gammad = (nu0).*((2.0.*1.38E-23.*T(i).*log(2.0))./(0.018.*3.0E8.*3.0E8./6.022E23)).^(0.5);\n    \n    y = (gammal./gammad).*((log(2.0)).^(0.5));\n    \n    x_on = ((nu_on-nu0)./gammad).*(log(2.0)).^(0.5);\n    \n    x_off = ((nu_off-nu0)./gammad).*(log(2.0)).^(0.5);\n    \n    %setting up Voigt convolution\n    stepsize = 1;\n    \n    t = [-200:1:199].*stepsize;\n    \n    t = repmat(t',1,length(x_on))';\n    \n    x_on = repmat(x_on,1,length(t));\n    \n    x_off = repmat(x_off,1,length(t));\n    \n    y = repmat(y,1,length(t));\n    \n    f_on = (exp(-t.^2.0))./(y.^2.0+(x_on-t).^2.0);\n    \n    f_off = (exp(-t.^2.0))./(y.^2.0+(x_off-t).^2.0);\n    \n    %Set the integration sum to zero to start\n    integral_on = 0.0;\n    \n    integral_off = 0.0;\n    \n    %Voigt integration\n    z_on = trapz(t(1,:),f_on,2);\n    \n    z_off =  trapz(t(1,:),f_off,2);\n    \n    integral_on = z_on;\n    \n    integral_off = z_off;\n    \n    %Calculate linestrength at temperature T\n    S = S0.*((T0./T(i)).^(1.5)).*exp(1.439.*E.*((1./T0)-(1./T(i))));\n    \n    %Calculate Doppler line-center cross section [cm^2]\n    K = (S./gammad).*(((log(2.0))./pi).^(0.5));\n    \n    %Calculate the Voigt profile\n    V_on = (y(1)/pi).*integral_on;\n    \n    V_off = (y(1)./pi).*integral_off;\n    \n    %Calculate the Voigt profile absorption cross section [cm^2]\n    sigmav_on = K.*V_on;\n    \n    sigmav_off = K.*V_off;\n    \n    %Sum contributions from all of the surrounding lines\n    sigma_on_total(i) = sum(sigmav_on);\n    \n    sigma_off_total(i) = sum(sigmav_off);\n    \nend;"("lambda"=w577, "lambda_off"=w580, "P0_mb"=w579, "T0_C"=w578, "Online"=w574) -> ("sigma_on_total"=→"sigma_on_total":dbl[], "sigma_off_total"=→"sigma_off_total":dbl[])  [unwired: 1 in, 1 out]
                  }
                }
              }
              frame #5 {
                w591 = 1
                # "normalization factor\nfrom 300 to 450m"
                # "OPTICAL DEPTH PLOT"
                # "new rainbow color bar display"
                # "Data Processing Far Channel"
                # "new rainbow color bar display"
                # "Calculating the range resolved water vapor number density and plotting"
                n454 = local read "sigma_off_total"() -> (w614:dbl[])
                n455 = local read "sigma_on_total"() -> (w611:dbl[])
                n456 = local read "On-Line  Smoothed"() -> (w589:dbl[])
                n457 = local read "Off-Line Smoothed"() -> (w588:dbl[])
                n458 = local read "Off-Line Smoothed 2"() -> (w612:dbl[])
                n459 = local read "On-Line Smoothed 2"() -> (w613:dbl[])
                n460 = script code="%Time averaging in seconds.  600 Seconds =10 minutes\ntemporal_average = 600;\n\n%Spatial averaging in bins.  2 bins = 150 meters\nspatial_average = 2;\n\n%Creating r and r+deltar vectors..this can also be acsomplished using the\n%diff command\np_oni = Online(:,1:size(Online,2)-1);\n\np_onii = Online(:,2:size(Online,2));\n\np_offi = Offline(:,1:size(Offline,2)-1);\n\np_offii = Offline(:,2:size(Offline,2));\n\nInside = (p_oni.*p_offii)./(p_onii.*p_offi);\n\ndel_cross = 1./(2.*(sigma_on_total(1:size(Online,2)-1)-sigma_off_total(1:size(Offline,2)-1)).*75*100);\n\ndel_cross(isinf(del_cross)) = 0;\n\n%Calculating Number density\nN = del_cross.*log(Inside);\n\n%Spatial smoothing of the profiles\nfilter1 = ones(1,2)./2;\n\nN_1 = N;\n\nN_1_avg = filter2(filter1,N_1);\n\nfilter1 = ones(1,10)./10;\n\nN_2 = N;\n\nN_2_avg = filter2(filter1,N_2);\n\nN_new = zeros(size(N,1),size(N,2));\n \n%Using different averaging windows for different altitudes \nN_avg=[N_1_avg(:,1:40)';N_2_avg(:,41:size(N,2))']';\n\n\nw = N_avg.*1e6.*18.015./6.022e23"("Online"=w613, "Offline"=w612, "sigma_on_total"=w611, "sigma_off_total"=w614) -> ("N_avg"=w615:cdb[], "w"=w624:cdb[])  [unwired: 1 in, 1 out]
                n461 = script code="%Time averaging in seconds.  600 Seconds = 10 minutes\ntemporal_average = 600;\n\n%Spatial averaging in bins.  2 bins = 150 meters\nspatial_average = 2;\n\n%Creating r and r+deltar vectors..this can also be acsomplished using the\n%diff command\np_oni = Online(:,1:size(Online,2)-1);\n\np_onii = Online(:,2:size(Online,2));\n\np_offi = Offline(:,1:size(Offline,2)-1);\n\np_offii = Offline(:,2:size(Offline,2));\n\nInside = (p_oni.*p_offii)./(p_onii.*p_offi);\n\ndel_cross = 1./(2.*(sigma_on_total(1:size(Online,2)-1)-sigma_off_total(1:size(Offline,2)-1)).*75*100);\n\ndel_cross(isinf(del_cross)) = 0;\n\n%Calculating Number density\nN = del_cross.*log(Inside);\n\n%Spatial smoothing of the profiles\nfilter1 = ones(1,2)./2;\n\nN_1 = N;\n\nN_1_avg = filter2(filter1,N_1);\n\nfilter1 = ones(1,10)./10;\n\nN_2 = N;\n\nN_2_avg = filter2(filter1,N_2);\n\nN_new = zeros(size(N,1),size(N,2));\n \n%Using different averaging windows for different altitudes \nN_avg=[N_1_avg(:,1:40)';N_2_avg(:,41:size(N,2))']';\n\n \nw = N_avg.*1e6.*18.015./6.022e23"("Online"=w589, "Offline"=w588, "sigma_on_total"=w611, "sigma_off_total"=w614) -> ("N_avg"=w620:cdb[], "w"=w621:cdb[])  [unwired: 1 in, 1 out]
                n462 = local read "Time Resolution Per Bin(ns)"() -> (w590:u32)
                n463 = local read "bins"() -> (w616:u32)
                n464 = local read "Altitude Array (km)"() -> (w586:dbl[])
                n465 = Build Array(w621, w624) -> (w627:cdb[][])
                n466 = To Double Precision Float(number=w590) -> (double precision float=w609:dbl)
                n467 = Reshape Array(w620, w591, w616) -> (w631:cdb[][])
                n468 = Reshape Array(w615, w591, w616) -> (w618:cdb[][])
                n469 = Multiply(x=0.15, y=w609) -> (x*y=w607:dbl)
                n470 = Build Array(w620, w615) -> (w625:cdb[][])
                n471 = Divide(x=300.0, y=w607) -> (x/y=w604:dbl)
                n472 = Divide(x=450.0, y=w607) -> (x/y=w603:dbl)
                n473 = Build Array(w586, w586) -> (w610:dbl[][])
                n474 = call "Convert to Dynamic Data5"("2D Array"=w627) -> ("Dynamic Data Type"=w626:dynamicdata)  [unwired: 3 in]
                n475 = call "Convert to Dynamic Data2"("2D Array"=w625) -> ("Dynamic Data Type"=w622:dynamicdata)  [unwired: 3 in]
                n476 = Divide(x=w631, y=1e+17) -> (x/y=→"Water Vapor Number Density":cdb[][])
                n477 = Divide(x=w618, y=1e+17) -> (x/y=→"Water Vapor Number Density 2":cdb[][])
                n478 = call "Convert to Dynamic Data6"("Array"=w586) -> ("Dynamic Data Type"=w587:dynamicdata)  [unwired: 3 in]
                n479 = To Long Integer(number=w604) -> (32bit integer=w602:i32)
                n480 = To Long Integer(number=w603) -> (32bit integer=w601:i32)
                n481 = call "Convert to Dynamic Data"("2D Array"=w610) -> ("Dynamic Data Type"=w623:dynamicdata)  [unwired: 3 in]
                n482 = call "Convert to Dynamic Data8"("2D Array"=w610) -> ("Dynamic Data Type"=w628:dynamicdata)  [unwired: 3 in]
                n483 = Decrement(x=w602) -> (x-1=w599:i32)
                n484 = Decrement(x=w601) -> (x-1=w600:i32)
                n485 = call "Build XY Graph"("Y Input"=w623, "X Input"=w622) -> ("XY Graph"=→"Water Vapor Number Density  2":cluster{"Y":dbl[], "Y":dbl[]}[])  [unwired: 3 in, 6 out]
                n486 = call "Build XY Graph3"("Y Input"=w628, "X Input"=w626) -> ("XY Graph"=→"Absolute Humidity":cluster{"Y":dbl[], "Y":dbl[]}[])  [unwired: 3 in, 6 out]
                n487 = Array Subset(array=w589, index=w599, length=w600) -> (w598:dbl[])
                n488 = Array Subset(array=w588, index=w599, length=w600) -> (w597:dbl[])
                n489 = call-poly <vilib>:"Mean.vi"("X"=w598) -> ("mean"=w596:dbl)  [unwired: 1 out]
                n490 = call-poly <vilib>:"Mean.vi"("X"=w597) -> ("mean"=w595:dbl)  [unwired: 1 out]
                n491 = Divide(x=w596, y=w595) -> (x/y=w594:dbl)
                n492 = Multiply(x=w588, y=w594) -> (x*y=w593:dbl[])
                n493 = Divide(x=w589, y=w593) -> (x/y=w592:dbl[])
                n494 = Natural Logarithm(1:w592) -> (0:w583:dbl[])
                n495 = Multiply(x=-1.0, y=w583) -> (x*y=w582:dbl[])
                n496 = call "Convert to Dynamic Data9"("Array"=w582) -> ("Dynamic Data Type"=w585:dynamicdata)  [unwired: 3 in]
                n497 = call "Build OD Plot"("Y Input"=w587, "X Input"=w585) -> ("XY Graph"=→"Optical Depth":cluster{"Y":dbl[], "Y":dbl[]}[])  [unwired: 3 in, 6 out]
              }
            }
          }
        }
        "L_Count" <- w126
      }
    }
  }
  n498 = case shown="True" w3 {
    frame False {
    }
    frame True {
      # "close data files"
      n499 = local read "NF_Off_Ref"() -> (w634:refnum<file>)
      n500 = local read "NF_On_Ref"() -> (w635:refnum<file>)
      n501 = local read "FF_Off_Ref"() -> (w636:refnum<file>)
      n502 = local read "FF_On_Ref"() -> (w637:refnum<file>)
      n503 = Close File(refnum=w637) -> ()  [unwired: 1 in, 2 out]
      n504 = Close File(refnum=w636) -> ()  [unwired: 1 in, 2 out]
      n505 = Close File(refnum=w635) -> ()  [unwired: 1 in, 2 out]
      n506 = Close File(refnum=w634) -> ()  [unwired: 1 in, 2 out]
    }
  }
  "FileHour" <- -1 ("FileHour")
  "DataOpen" <- FALSE
